vi "RF Scope Control.vi"() -> ()   [LabVIEW 2020]
uses:
  Sub VIs/Scope/Typedefs/Scope Control References Control.ctl
  Sub VIs/Power Supply/Typedefs/Power Supply Models.ctl
  Sub VIs/Settings/Typedefs/Save Settings Control References Control.ctl
  Sub VIs/DMM/Typedefs/DMM Control Variable References.ctl
  Sub VIs/Power Supply/Typedefs/PS Control Variable References.ctl
  Sub VIs/Measurements/Typedefs/Experiment Config Control.ctl
  Sub VIs/Measurements/Typedefs/Measurement Config.ctl
  Sub VIs/Settings/Typedefs/Save settings cluster.ctl
  Sub VIs/Global Vars.vi
  <vilib>/Utility/file.llb/Write Delimited Spreadsheet (string).vi
panel:
  in  "Scope Control References":T1
  in  "PS Reconnecting 2":bool
  in  "DMM Reconnecting 2":bool
  out "Headers":string[](array[string])
  in  "Scope Reconnecting":bool
  in  "PS Reconnecting":bool
  in  "DMM Reconnecting":bool
  in  "Tab Control 2":T2(tab)
  in  "Scope Config on Startup":enum16{"PC->Scope", "Scope->PC"}(ring)=enum."Scope->PC"
  in  "Scope Model":u16(ring)=1 items=["Tek TDS 684A/B/C", "Tek TDS 694C", "Tek TDS 744/A", "Tek TDS 754A/C/D", "Tek TDS 784A/C/D"]
  in  "Disconnect Scope":bool
  in  "Connect Scope":bool
  in  "Reset Settings":bool
  out "Connected Scope":string
  in  "Scope Address":refnum<visa-resource-name>
  out "Scope Connected":bool
  in  "Vertical Scale":u16(ring)=6 items=["1mV", "2mV", "5mV", "10mV", "20mV", "50mV", "100mV", "200mV", "500mV", "1V", "2V", "5V", "10V"]
  in  "Trigger Coupling":i32(ring)=1 items=["main trigger", "DC", "noise reject"]
  in  "Trigger Slope":i32(ring) items=["Positive", "Negative"]
  in  "Horizontle Scale":i32(ring)=19 items=["100ps/div", "200ps/div", "500ps/div", "1ns/div", "2ns/div", "5ns/div", "10ns/div", "20ns/div", "50ns/div", "100ns/div", "200ns/div", "500ns/div", "1µs/div", "2µs/div", "5µs/div", "10µs/div", "20µs/div", "50µs/div", "100µs/div", "200µs/div", "500µs/div", "1ms/div", "2ms/div", "5ms/div", "10ms/div", "20ms/div", "50ms/div", "100ms/div", "200ms/div", "500ms/div", "1s/div", "2s/div", "5s/div", "10s/div"]
  in  "Horizontle Trace Display":i32(ring)=1 items=["Main Only", "Intensified", "Delayed Only"]
  in  "Record Sample Length":i32(ring)=2 items=["500 points", "1000 points", "2500 points", "5000 points", "15000 points", "50000 points", "75000 points", "100000 points", "130000 points", "250000 points", "500000 points"]
  in  "Trigger Source":u16(ring) items=["Ch. 01", "Ch 02", "Ch. 03", "Ch. 04", "Aux"]
  in  "Trigger Level (V)":dbl
  in  "Trigger Type":u16(ring)=1 items=["Auto", "Normal"]
  in  "Coupling":u16(ring)=1 items=["AC", "DC", "Ground"]
  in  "Bandwidth":u16(ring)=2 items=["20 MHz", "250 MHz", "Full"]
  in  "Input Impedance":u16(ring) items=["50 Ohm", "1 MOhm"]
  in  "Waveform Source":u16(ring) items=["Ch. 01", "Ch 02", "Ch. 03", "Ch. 04"]
  in  "Repetitive Signal":bool
  in  "Power Supply Model 2":T3=enum."Keithley 24XX"
  in  "Power Supply Config on Startup 2":enum16{"PC->Power Supply", "Power Supply->PC"}(ring)=enum."Power Supply->PC"
  out "PS Connected 2":bool
  in  "Disconnect PS 2":bool
  in  "Connect PS 2":bool
  in  "ResetPS Settings 2":bool=TRUE
  out "Connected Power Supply 2":string
  in  "Power Supply Address 2":refnum<visa-resource-name>="GPIB0::5::INSTR"
  in  "Power Supply Config on Startup":enum16{"PC->Power Supply", "Power Supply->PC"}(ring)=enum."Power Supply->PC"
  out "PS Connected":bool
  in  "Disconnect PS":bool
  in  "Connect PS":bool
  in  "ResetPS Settings":bool=TRUE
  out "Connected Power Supply":string
  in  "Power Supply Address":refnum<visa-resource-name>="GPIB0::5::INSTR"
  in  "Power Supply Model":T3=enum."Keithley 24XX"
  out "Output Current 2":dbl
  in  "Filter Mode 2":u16(ring) items=["Output Filter Disabled", "Filter 1 On", "Filter 2 On"]
  in  "HV Out 2":bool
  in  "Trip Mode 2":u16(ring) items=["Manual Trip", "Auto Trip"]
  in  "Current Trip 2":dbl=0.005 min=0.0 max=0.005 step=1e-06 format="%.6f"
  in  "Voltage Limit 2":dbl=1000.0
  in  "Current Limit 2":dbl=0.0049 min=0.0 max=0.005 step=1e-06 format="%.6f"
  in  "Voltage Level 2":sgl
  out "Output Voltage 2":dbl
  out "Output Current":dbl
  in  "Filter Mode":u16(ring) items=["Output Filter Disabled", "Filter 1 On", "Filter 2 On"]
  in  "HV Out":bool
  in  "Trip Mode":u16(ring) items=["Manual Trip", "Auto Trip"]
  in  "Current Trip":dbl=0.005 min=0.0 max=0.005 step=1e-06 format="%.6f"
  in  "Voltage Limit":dbl=1000.0
  in  "Current Limit":dbl=0.0049 min=0.0 max=0.005 step=1e-06 format="%.6f"
  in  "Voltage Level":sgl
  out "Output Voltage":dbl
  in  "Identify DMM 2":bool
  in  "Identify DMM":bool
  in  "DMM Config on Startup 2":enum16{"PC->DMM", "DMM->PC"}(ring)=enum."DMM->PC"
  out "DMM Connected 2":bool
  in  "DMM Model 2":u16(ring) items=["Agilent 34405A"]
  in  "Disconnect DMM 2":bool
  in  "Connect DMM 2":bool
  in  "DMM Reset 2":bool
  out "Connected DMM 2":string
  in  "DMM Address 2":refnum<visa-resource-name>="GPIB0::5::INSTR"
  in  "DMM Config on Startup":enum16{"PC->DMM", "DMM->PC"}(ring)=enum."DMM->PC"
  out "DMM Connected":bool
  in  "DMM Model":u16(ring) items=["Agilent 34405A"]
  in  "Disconnect DMM":bool
  in  "Connect DMM":bool
  in  "DMM Reset":bool
  out "Connected DMM":string
  in  "DMM Address":refnum<visa-resource-name>="GPIB0::5::INSTR"
  out "DMM Measurement 2":dbl
  in  "DMM Measurement Type 2":i32(ring) items=["DC Volts", "AC Volts", "DC Current", "AC Current", "2-Wire Resistance", "Frequency", "Temperature", "Capacitance", "Continuity", "Diode", "4-Wire Resistance", "2nd DC Volts", "2nd AC Volts", "2nd DC Current", "2nd AC Current", "2nd Frequency"]
  out "DMM Measurement":dbl
  in  "DMM Measurement Type":i32(ring) items=["DC Volts", "AC Volts", "DC Current", "AC Current", "2-Wire Resistance", "Frequency", "Temperature", "Capacitance", "Continuity", "Diode", "4-Wire Resistance", "2nd DC Volts", "2nd AC Volts", "2nd DC Current", "2nd AC Current", "2nd Frequency"]
  in  "Delimiter":u8(ring)=44 items=["Comma"=44, "Tab"=9, "Semicolon"=59]
  out "Traces Saved":u64
  out "Filename":string
  in  "Start Measurement":bool
  in  "Stop Measurement":bool
  in  "Traces to Acquire":u64=100 min=1 step=1
  in  "Measurement Mode":T4(ring)
  out "Full File Path":path
  out "Measurements Running":bool
  out "Scope Trace":waveform(dbl)(graph)
  in  "Exit":bool
  # "Diode Power Supply"
  # "Amplifier Power Supply"
  # "HV ON"
  # "HV ON"
  # "HV OFF"
  # "HV OFF"
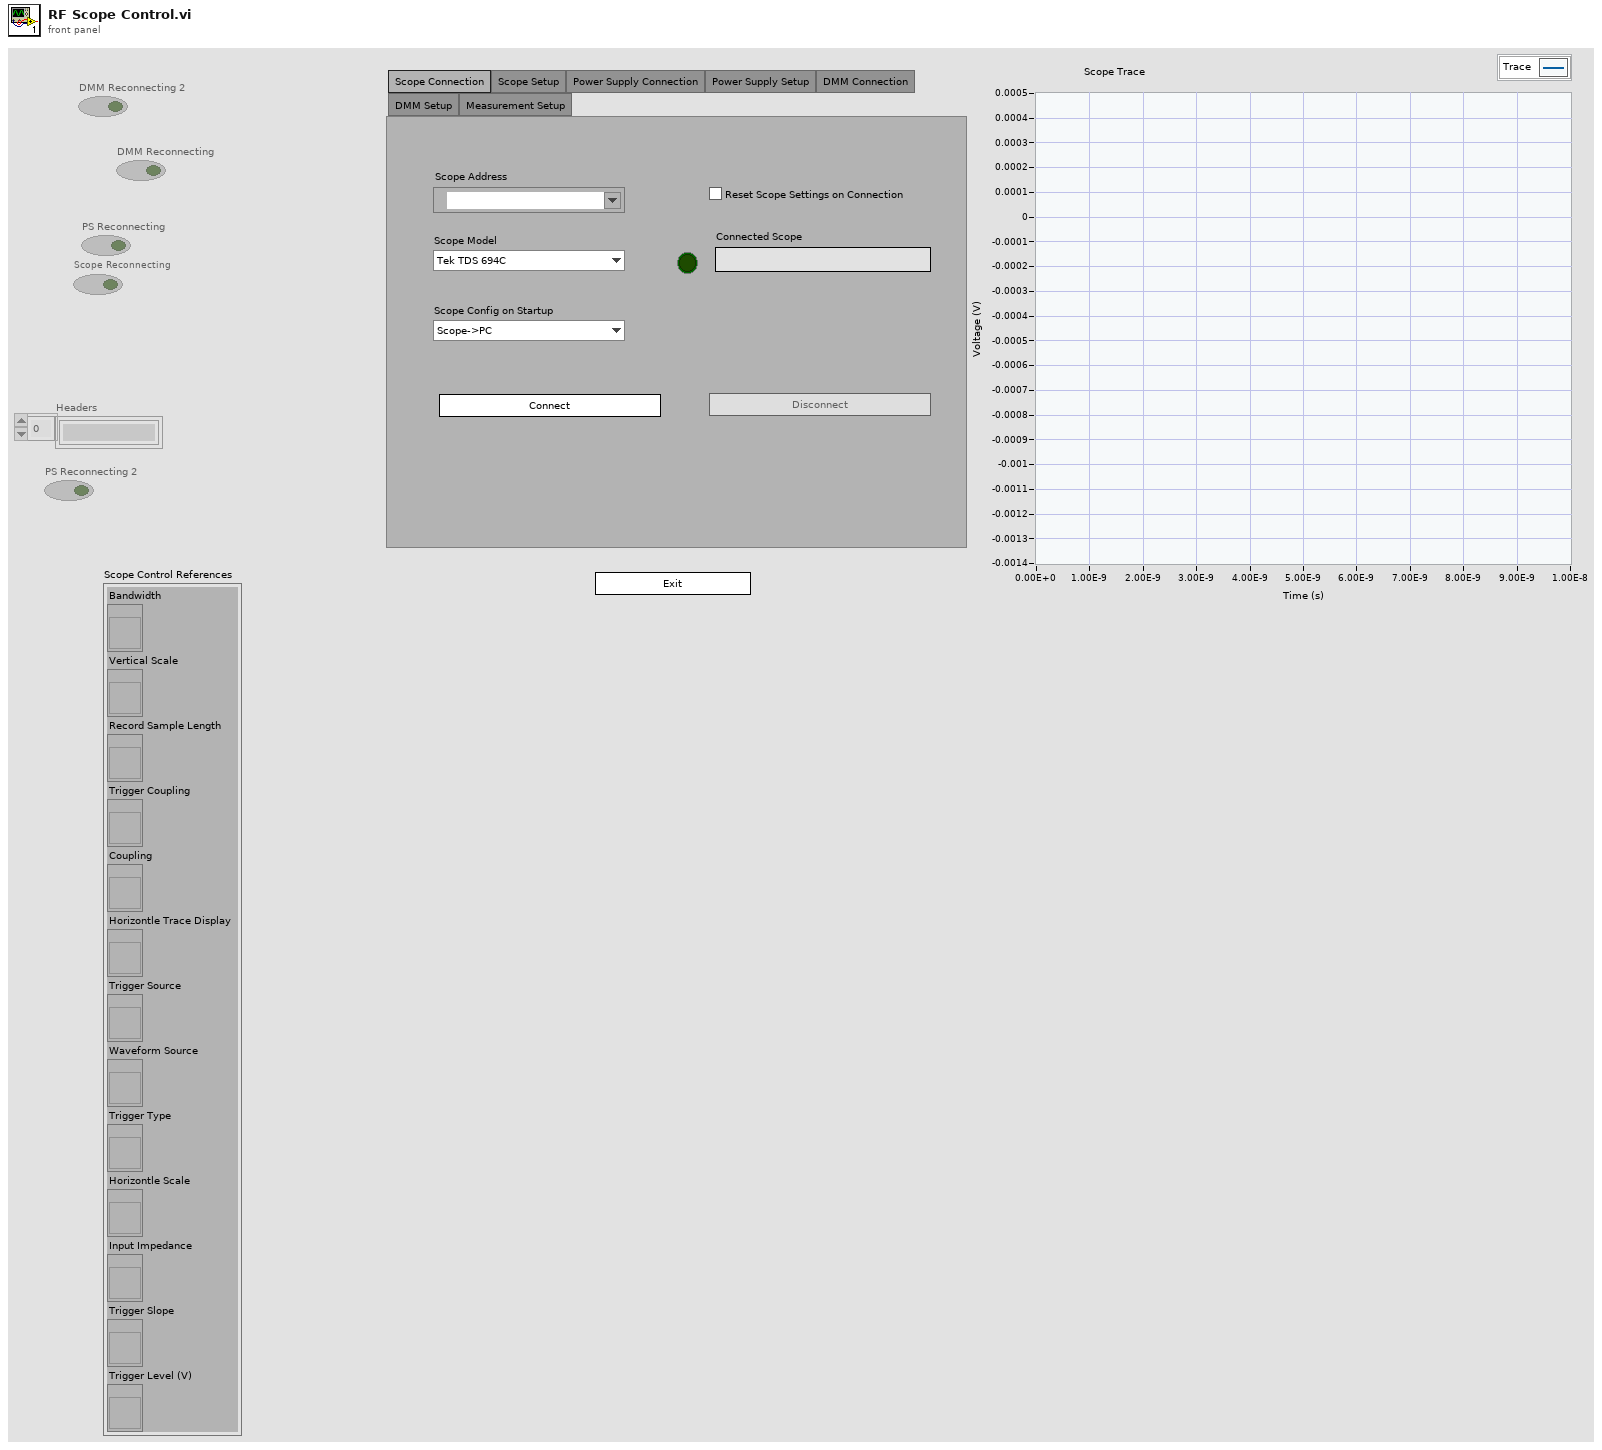
[diagram p1: front panel]
types:
  T1 = typedef "Scope Control References Control.ctl" = cluster{"Bandwidth":refnum<vi>, "Vertical Scale":refnum<vi>, "Record Sample Length":refnum<vi>, "Trigger Coupling":refnum<vi>, "Coupling":refnum<vi>, "Horizontle Trace Display":refnum<vi>, "Trigger Source":refnum<vi>, "Waveform Source":refnum<vi>, "Trigger Type":refnum<vi>, "Horizontle Scale":refnum<vi>, "Input Impedance":refnum<vi>, "Trigger Slope":refnum<vi>, "Trigger Level (V)":refnum<vi>}
  T2 = enum32{"Scope Connection", "Scope Setup", "Power Supply Connection", "Power Supply Setup", "DMM Connection", "DMM Setup", "Measurement Setup"}
  T3 = typedef "Power Supply Models.ctl" = enum16{"Keithley 248", "Keithley 237", "Keithley 24XX", "HP/Agilent 6XXX"}
  T4 = enum16{"Store All Traces in Single File", "Store Average/Std. Dev. for each Point", "Store All Traces in Separate Files"}
  T5 = typedef "PS Control Variable References.ctl" = cluster{"Exit":refnum<vi>, "Power Supply Address":refnum<vi>, "ResetPS Settings":refnum<vi>, "Power Supply Model":refnum<vi>, "PS Connected":refnum<vi>, "Connected Power Supply":refnum<vi>, "Power Supply Config on Startup":refnum<vi>, "Connect PS":refnum<vi>, "Disconnect PS":refnum<vi>, "Voltage Level":refnum<vi>, "Voltage Limit":refnum<vi>, "Current Trip":refnum<vi>, "Current Limit":refnum<vi>, "Trip Mode":refnum<vi>, "Filter Mode":refnum<vi>, "HV Out":refnum<vi>, "Output Voltage":refnum<vi>, "Output Current":refnum<vi>, "PS Reconnecting":refnum<vi>, "semaphore":T6, "Offline Controls":refnum<vi>[], "Online Controls":refnum<vi>[]}
  T6 = typedef "Semaphore RefNum" = refnum<k1>
  T7 = typedef "DMM Control Variable References.ctl" = cluster{"Exit":refnum<vi>, "DMM Connected":refnum<vi>, "DMM Reconnecting":refnum<vi>, "DMM Address":refnum<vi>, "DMM Model":refnum<vi>, "DMM Measurement":refnum<vi>, "Wait on Other Threads":refnum<vi>, "DMM Reset":refnum<vi>, "DMM Config on Startup":refnum<vi>, "DMM Measurement Type":refnum<vi>, "Disconnect DMM":refnum<vi>, "Connect DMM":refnum<vi>, "Identify DMM":refnum<vi>, "Connected DMM":refnum<vi>, "semaphore":T6, "Online Controls":refnum<vi>[], "Offline Controls":refnum<vi>[]}
  T8 = typedef "Save Settings Control References Control.ctl" = cluster{"DMM Config on Startup":refnum<vi>, "Power Supply Config on Startup":refnum<vi>, "Repetitive Signal":refnum<vi>, "Scope Address":refnum<vi>, "Reset Settings":refnum<vi>, "Scope Model":refnum<vi>, "Scope Config on Startup":refnum<vi>, "Waveform Source":refnum<vi>, "Input Impedance":refnum<vi>, "Bandwidth":refnum<vi>, "Coupling":refnum<vi>, "Horizontle Trace Display":refnum<vi>, "Horizontle Scale":refnum<vi>, "Record Sample Length":refnum<vi>, "Trigger Source":refnum<vi>, "Trigger Level (V)":refnum<vi>, "Trigger Slope":refnum<vi>, "Trigger Coupling":refnum<vi>, "Vertical Scale":refnum<vi>, "Trigger Type":refnum<vi>, "Power Supply Address":refnum<vi>, "ResetPS Settings":refnum<vi>, "Voltage Level":refnum<vi>, "Voltage Limit":refnum<vi>, "Current Trip":refnum<vi>, "Current Limit":refnum<vi>, "Trip Mode":refnum<vi>, "Filter Mode":refnum<vi>, "DMM Address":refnum<vi>, "DMM Reset":refnum<vi>, "DMM Model":refnum<vi>, "DMM Measurement Type":refnum<vi>, "Traces to Acquire":refnum<vi>, "Measurement Mode":refnum<vi>, "Power Supply Model":refnum<vi>}
  T9 = enum8{"Enabled", "Disabled", "Disabled and Grayed Out"}
  T10 = typedef "Save settings cluster.ctl" = cluster{"Bandwidth":u16, "Coupling":u16, "Current Limit":dbl, "Current Trip":dbl, "DMM Address":refnum<visa-resource-name>, "DMM Measurement Type":i32, "DMM Model":u16, "DMM Reset":bool, "Filter Mode":u16, "Horizontle Scale":i32, "Horizontle Trace Display":i32, "Input Impedance":u16, "Power Supply Address":refnum<visa-resource-name>, "Record Sample Length":i32, "Reset Settings":bool, "ResetPS Settings":bool, "Scope Address":refnum<visa-resource-name>, "Scope Config on Startup":u16, "Traces to Acquire":u64, "Trigger Coupling":i32, "Trigger Level (V)":dbl, "Trigger Slope":i32, "Trigger Source":u16, "Trigger Type":u16, "Trip Mode":u16, "Vertical Scale":u16, "Voltage Level":sgl, "Voltage Limit":dbl, "Waveform Source":u16, "Scope Model":u16, "DMM Config on Startup":enum16{"PC->DMM", "DMM->PC"}, "Power Supply Config on Startup":enum16{"PC->Power Supply", "Power Supply->PC"}, "Repetitive Signal":bool, "Measurement Mode":enum16{"Store All Traces in Single File", "Store Average/Std. Dev. for each Point", "Store All Traces in Separate Files"}, "Power Supply Model":T3}
  T11 = typedef "Measurement Config.ctl" = cluster{"Measurement Mode":enum16{"Store All Traces in Single File", "Store Average/Std. Dev. for each Point", "Store All Traces in Separate Files"}, "Full File Path":path, "Filename":string, "Delimiter":string, "Headers":string[]}
  T12 = typedef "Experiment Config Control.ctl" = cluster{"PS Connected":bool, "DMM Connected":bool, "DMM Connected 2":bool, "PS HV On":bool}
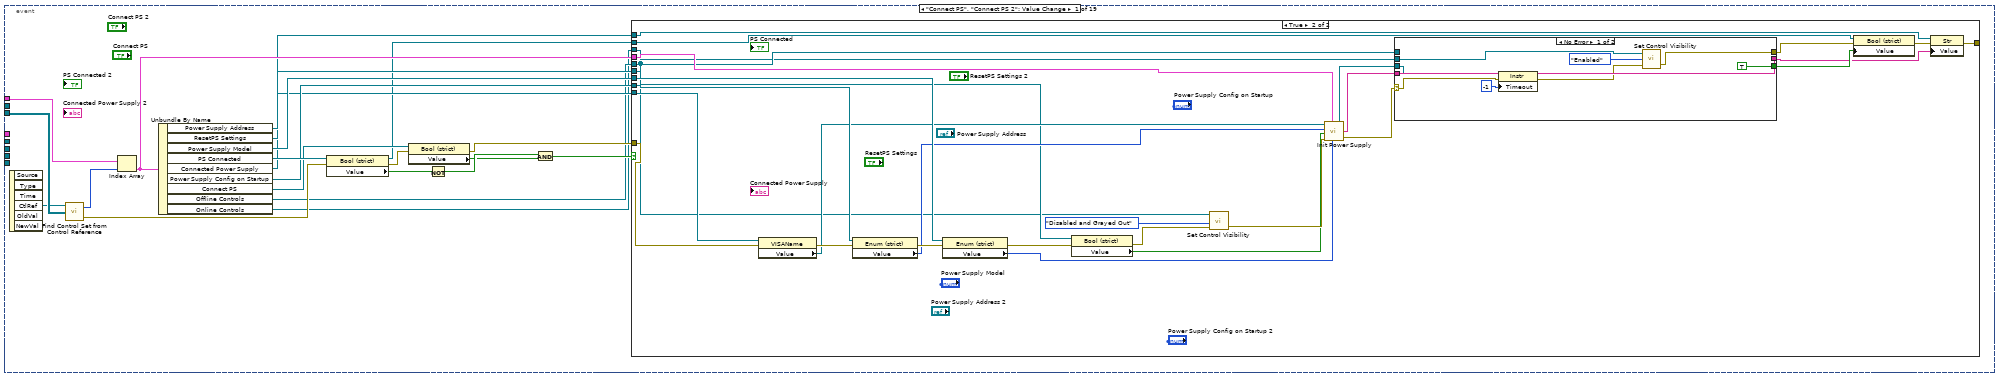
[diagram p14: hidden frame]
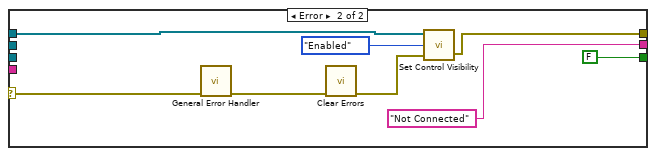
[diagram p16: hidden frame]
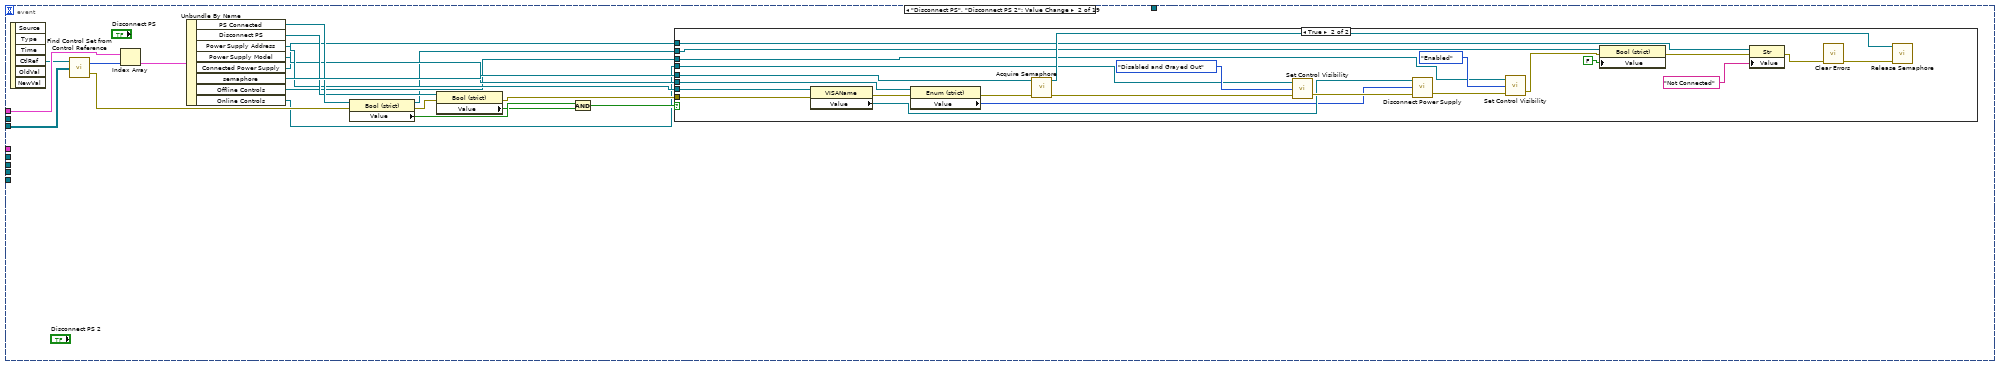
[diagram p17: hidden frame]
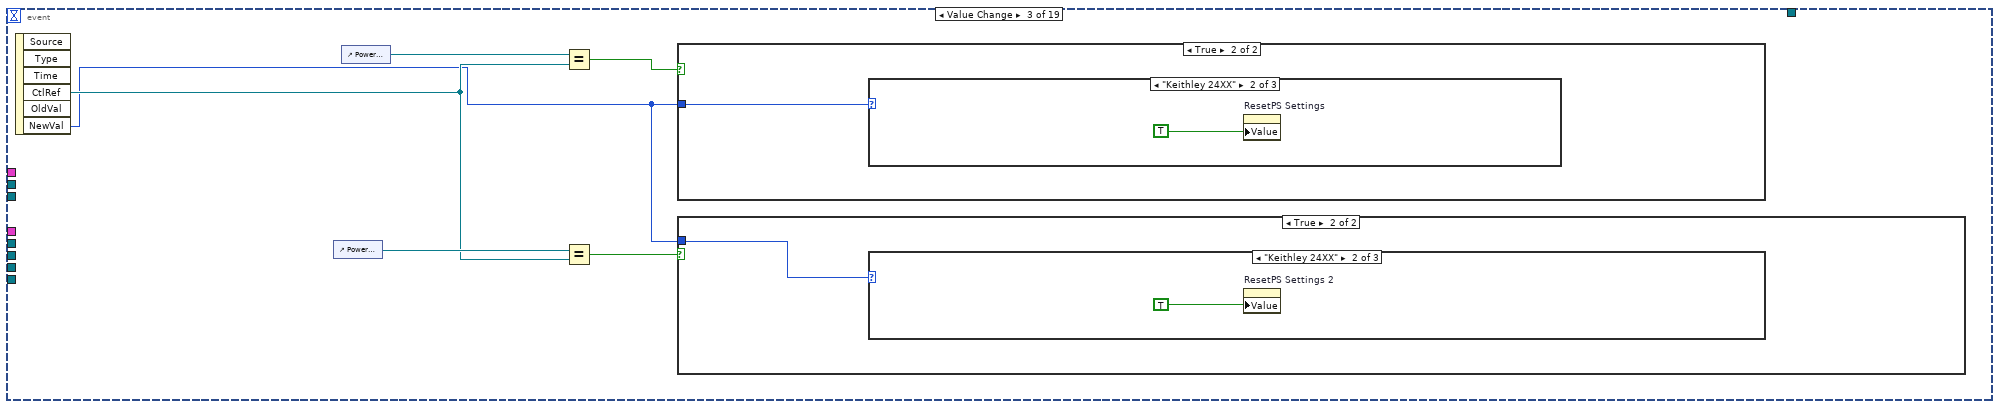
[diagram p19: hidden frame]
diagram:
  w31 = T5 {"Exit"=refnum, "Power Supply Address"=refnum, "ResetPS Settings"=refnum, "Power Supply Model"=refnum, "PS Connected"=refnum, "Connected Power Supply"=refnum, "Power Supply Config on Startup"=refnum, "Connect PS"=refnum, "Disconnect PS"=refnum, "Voltage Level"=refnum, "Voltage Limit"=refnum, "Current Trip"=refnum, "Current Limit"=refnum, "Trip Mode"=refnum, "Filter Mode"=refnum, "HV Out"=refnum, "Output Voltage"=refnum, "Output Current"=refnum, "PS Reconnecting"=refnum, "semaphore"=refnum, "Offline Controls"=[], "Online Controls"=[]}  # PS Control References Array
  w78 = T7 {"Exit"=refnum, "DMM Connected"=refnum, "DMM Reconnecting"=refnum, "DMM Address"=refnum, "DMM Model"=refnum, "DMM Measurement"=refnum, "Wait on Other Threads"=refnum, "DMM Reset"=refnum, "DMM Config on Startup"=refnum, "DMM Measurement Type"=refnum, "Disconnect DMM"=refnum, "Connect DMM"=refnum, "Identify DMM"=refnum, "Connected DMM"=refnum, "semaphore"=refnum, "Online Controls"=[], "Offline Controls"=[]}  # DMM Control References Array
  w112 = T8 {"DMM Config on Startup"=refnum, "Power Supply Config on Startup"=refnum, "Repetitive Signal"=refnum, "Scope Address"=refnum, "Reset Settings"=refnum, "Scope Model"=refnum, "Scope Config on Startup"=refnum, "Waveform Source"=refnum, "Input Impedance"=refnum, "Bandwidth"=refnum, "Coupling"=refnum, "Horizontle Trace Display"=refnum, "Horizontle Scale"=refnum, "Record Sample Length"=refnum, "Trigger Source"=refnum, "Trigger Level (V)"=refnum, "Trigger Slope"=refnum, "Trigger Coupling"=refnum, "Vertical Scale"=refnum, "Trigger Type"=refnum, "Power Supply Address"=refnum, "ResetPS Settings"=refnum, "Voltage Level"=refnum, "Voltage Limit"=refnum, "Current Trip"=refnum, "Current Limit"=refnum, "Trip Mode"=refnum, "Filter Mode"=refnum, "DMM Address"=refnum, "DMM Reset"=refnum, "DMM Model"=refnum, "DMM Measurement Type"=refnum, "Traces to Acquire"=refnum, "Measurement Mode"=refnum, "Power Supply Model"=refnum}  # Controls References
  n1 = control-ref of="Power Supply Config on Startup"() -> (w51:refnum<vi>)
  n2 = control-ref of="DMM Measurement Type"() -> (w83:refnum<vi>)
  n3 = control-ref of="Scope Config on Startup"() -> (w96:refnum<vi>)
  n4 = control-ref of="DMM Config on Startup"() -> (w84:refnum<vi>)
  n5 = control-ref of="Horizontle Trace Display"() -> (w102:refnum<vi>)
  n6 = control-ref of="Power Supply Address"() -> (w53:refnum<vi>)
  n7 = control-ref of="DMM Address"() -> (w88:refnum<vi>)
  n8 = control-ref of="Scope Address"() -> (w109:refnum<vi>)
  n9 = control-ref of="Record Sample Length"() -> (w101:refnum<vi>)
  n10 = control-ref of="Power Supply Model"() -> (w90:refnum<vi>)
  n11 = control-ref of="Power Supply Model"() -> (w50:refnum<vi>)
  n12 = control-ref of="Measurement Mode"() -> (w97:refnum<vi>)
  n13 = control-ref of="Disconnect Scope"() -> (w119:refnum<vi>)
  n14 = control-ref of="Waveform Source"() -> (w107:refnum<vi>)
  n15 = control-ref of="Input Impedance"() -> (w91:refnum<vi>)
  n16 = control-ref of="Traces to Acquire"() -> (w98:refnum<vi>)
  n17 = control-ref of="Trigger Coupling"() -> (w100:refnum<vi>)
  n18 = control-ref of="ResetPS Settings"() -> (w52:refnum<vi>)
  n19 = control-ref of="Repetitive Signal"() -> (w108:refnum<vi>)
  n20 = control-ref of="Horizontle Scale"() -> (w93:refnum<vi>)
  n21 = control-ref of="Trigger Level (V)"() -> (w104:refnum<vi>)
  n22 = control-ref of="Connect Scope"() -> (w118:refnum<vi>)
  n23 = control-ref of="Connect DMM"() -> (w85:refnum<vi>)
  n24 = control-ref of="Trigger Source"() -> (w103:refnum<vi>)
  n25 = control-ref of="Disconnect PS"() -> (w8:refnum<vi>)
  n26 = control-ref of="Reset Settings"() -> (w110:refnum<vi>)
  n27 = control-ref of="Voltage Level"() -> (w47:refnum<vi>)
  n28 = control-ref of="Voltage Limit"() -> (w48:refnum<vi>)
  n29 = control-ref of="Current Limit"() -> (w45:refnum<vi>)
  n30 = control-ref of="Trigger Slope"() -> (w94:refnum<vi>)
  n31 = control-ref of="Vertical Scale"() -> (w99:refnum<vi>)
  n32 = control-ref of="Scope Model"() -> (w95:refnum<vi>)
  n33 = control-ref of="DMM Model"() -> (w87:refnum<vi>)
  n34 = control-ref of="Trigger Type"() -> (w105:refnum<vi>)
  n35 = control-ref of="Current Trip"() -> (w46:refnum<vi>)
  n36 = control-ref of="Connect PS"() -> (w54:refnum<vi>)
  n37 = control-ref of="Filter Mode"() -> (w43:refnum<vi>)
  n38 = control-ref of="DMM Reset"() -> (w89:refnum<vi>)
  n39 = control-ref of="HV Out"() -> (w49:refnum<vi>)
  n40 = control-ref of="Bandwidth"() -> (w92:refnum<vi>)
  n41 = control-ref of="Trip Mode"() -> (w44:refnum<vi>)
  n42 = control-ref of="Coupling"() -> (w106:refnum<vi>)
  n43 = control-ref of="Stop Measurement"() -> (w2:refnum<vi>)
  n44 = Bundle By Name(cluster=w112, "DMM Config on Startup"=w84, "Power Supply Config on Startup"=w51, "Repetitive Signal"=w108, "Scope Address"=w109, "Reset Settings"=w110, "Scope Model"=w95, "Scope Config on Startup"=w96, "Waveform Source"=w107, "Input Impedance"=w91, "Bandwidth"=w92, "Coupling"=w106, "Horizontle Trace Display"=w102, "Horizontle Scale"=w93, "Record Sample Length"=w101, "Trigger Source"=w103, "Trigger Level (V)"=w104, "Trigger Slope"=w94, "Trigger Coupling"=w100, "Vertical Scale"=w99, "Trigger Type"=w105, "Power Supply Address"=w53, "ResetPS Settings"=w52, "Power Supply Model"=w50, "Voltage Level"=w47, "Voltage Limit"=w48, "Current Trip"=w46, "Current Limit"=w45, "Trip Mode"=w44, "Filter Mode"=w43, "DMM Address"=w88, "DMM Reset"=w89, "DMM Model"=w87, "DMM Measurement Type"=w83, "Traces to Acquire"=w98, "Measurement Mode"=w97) -> (w111:T8)
  n45 = Build Array(w119, w107, w106, w105, w103, w104, w94, w102, w101, w100, w93, w99, w108, w92, w91) -> (w130:refnum<vi>[])
  n46 = Build Array(w8, w49, w43, w44, w45, w46, w48, w47) -> (w33:refnum<vi>[])
  n47 = Build Array(w53, w52, w54, w90, w51) -> (w34:refnum<vi>[])
  n48 = Build Array(w88, w89, w85, w84, w87) -> (w62:refnum<vi>[])
  n49 = Build Array(w110, w109, w118, w95, w96) -> (w133:refnum<vi>[])
  n50 = Build Array(w2) -> (w1:refnum<vi>[])
  n51 = Current VI's Path() -> (path=w115:path)
  n52 = call "Recall Settings From XML File.vi"("Controls References"=w111, "Settings File Name"="config.xml", "Settings File Path"=w115) -> ("error out"=w113:errorcluster)  [unwired: 2 in]
  n53 = call <vilib>:"Clear Errors.vi"("error in (no error)"=w113) -> ("error out"=w60:errorcluster)  [unwired: 5 in, 1 out]
  n54 = control-ref of="Disconnect DMM"() -> (w86:refnum<vi>)
  n55 = control-ref of="Identify DMM"() -> (w82:refnum<vi>)
  n56 = Build Array(w86, w83, w82) -> (w61:refnum<vi>[])
  n57 = call <vilib>:"Obtain Semaphore Reference.vi"("error in (no error)"=w60, "name (unnamed)"="DMM Semaphore") -> ("error out"=w137:errorcluster, "semaphore"=w63:T6)  [unwired: 3 in, 1 out]
  n58 = control-ref of="DMM Measurement Type 2"() -> (w72:refnum<vi>)
  n59 = control-ref of="DMM Config on Startup 2"() -> (w76:refnum<vi>)
  n60 = control-ref of="DMM Address 2"() -> (w74:refnum<vi>)
  n61 = control-ref of="DMM Reconnecting 2"() -> (w37:refnum<vi>)
  n62 = control-ref of="DMM Reconnecting"() -> (w80:refnum<vi>)
  n63 = control-ref of="DMM Measurement"() -> (w79:refnum<vi>)
  n64 = control-ref of="Disconnect DMM 2"() -> (w70:refnum<vi>)
  n65 = control-ref of="DMM Connected 2"() -> (w30:refnum<vi>)
  n66 = control-ref of="Start Measurement"() -> (w38:refnum<vi>)
  n67 = control-ref of="PS Reconnecting 2"() -> (w15:refnum<vi>)
  n68 = control-ref of="Connected DMM"() -> (w67:refnum<vi>)
  n69 = control-ref of="DMM Connected"() -> (w81:refnum<vi>)
  n70 = control-ref of="PS Reconnecting"() -> (w35:refnum<vi>)
  n71 = control-ref of="Connect DMM 2"() -> (w73:refnum<vi>)
  n72 = control-ref of="Identify DMM 2"() -> (w71:refnum<vi>)
  n73 = control-ref of="DMM Model 2"() -> (w68:refnum<vi>)
  n74 = control-ref of="PS Connected"() -> (w42:refnum<vi>)
  n75 = control-ref of="DMM Reset 2"() -> (w75:refnum<vi>)
  n76 = control-ref of="HV Out 2"() -> (w18:refnum<vi>)
  n77 = control-ref of="Exit"() -> (w77:refnum<vi>)
  n78 = control-ref of="Measurements Running"() -> (w6:refnum<vi>)
  n79 = control-ref of="Scope Connected"() -> (w7:refnum<vi>)
  n80 = control-ref of="Delimiter"() -> (w4:refnum<vi>)
  n81 = Bundle By Name(cluster=w78, "Exit"=w77, "DMM Connected"=w81, "DMM Reconnecting"=w80, "DMM Address"=w88, "DMM Model"=w87, "DMM Measurement"=w79, "Identify DMM"=w82, "DMM Reset"=w89, "DMM Config on Startup"=w84, "DMM Measurement Type"=w83, "Disconnect DMM"=w86, "Connect DMM"=w85, "Connected DMM"=w67, "semaphore"=w63, "Online Controls"=w61, "Offline Controls"=w62) -> (w64:T7)
  n82 = Build Array(w74, w75, w76, w73, w68) -> (w55:refnum<vi>[])
  n83 = Build Array(w70, w72, w71) -> (w56:refnum<vi>[])
  n84 = Build Array(w98, w38, w97, w4) -> (w3:refnum<vi>[])
  n85 = call <vilib>:"Obtain Semaphore Reference.vi"("error in (no error)"=w137, "name (unnamed)"="DMM 2 Semaphore") -> ("error out"=w136:errorcluster, "semaphore"=w57:T6)  [unwired: 3 in, 1 out]
  n86 = global write "Global Vars.vi" "DMM 1 Controls"(w64) -> ()
  n87 = control-ref of="DMM Measurement 2"() -> (w69:refnum<vi>)
  n88 = control-ref of="Connected DMM 2"() -> (w66:refnum<vi>)
  n89 = Bundle By Name(cluster=w78, "Exit"=w77, "DMM Connected"=w30, "DMM Reconnecting"=w37, "DMM Address"=w74, "DMM Model"=w68, "DMM Measurement"=w69, "Identify DMM"=w71, "DMM Reset"=w75, "DMM Config on Startup"=w76, "DMM Measurement Type"=w72, "Disconnect DMM"=w70, "Connect DMM"=w73, "Connected DMM"=w66, "semaphore"=w57, "Online Controls"=w56, "Offline Controls"=w55) -> (w65:T7)
  n90 = call <vilib>:"Obtain Semaphore Reference.vi"("error in (no error)"=w136, "name (unnamed)"="Scope Semaphore") -> ("error out"=w141:errorcluster, "semaphore"=w140:T6)  [unwired: 3 in, 1 out]
  n91 = global write "Global Vars.vi" "DMM 2 Controls"(w65) -> ()
  n92 = control-ref of="Power Supply Config on Startup 2"() -> (w25:refnum<vi>)
  n93 = control-ref of="Power Supply Address 2"() -> (w29:refnum<vi>)
  n94 = control-ref of="Power Supply Model 2"() -> (w27:refnum<vi>)
  n95 = call <vilib>:"Obtain Semaphore Reference.vi"("error in (no error)"=w141, "name (unnamed)"="PS Semaphore") -> ("error out"=w127:errorcluster, "semaphore"=w40:T6)  [unwired: 3 in, 1 out]
  n96 = control-ref of="ResetPS Settings 2"() -> (w28:refnum<vi>)
  n97 = control-ref of="Connect PS 2"() -> (w10:refnum<vi>)
  n98 = control-ref of="Connected Power Supply 2"() -> (w26:refnum<vi>)
  n99 = control-ref of="Connected Power Supply"() -> (w41:refnum<vi>)
  n100 = Build Array(w29, w28, w27, w25, w10) -> (w11:refnum<vi>[])
  n101 = control-ref of="Connected Scope"() -> (w121:refnum<vi>)
  n102 = control-ref of="Disconnect PS 2"() -> (w9:refnum<vi>)
  n103 = control-ref of="Output Voltage"() -> (w39:refnum<vi>)
  n104 = control-ref of="Output Current"() -> (w36:refnum<vi>)
  n105 = control-ref of="Voltage Level 2"() -> (w24:refnum<vi>)
  n106 = control-ref of="Voltage Limit 2"() -> (w23:refnum<vi>)
  n107 = control-ref of="Current Limit 2"() -> (w21:refnum<vi>)
  n108 = control-ref of="Current Trip 2"() -> (w22:refnum<vi>)
  n109 = control-ref of="Filter Mode 2"() -> (w19:refnum<vi>)
  n110 = control-ref of="Trip Mode 2"() -> (w20:refnum<vi>)
  n111 = Bundle By Name(cluster=w31, "Exit"=w30, "Power Supply Address"=w53, "ResetPS Settings"=w52, "Power Supply Model"=w50, "PS Connected"=w42, "Connected Power Supply"=w41, "Power Supply Config on Startup"=w51, "Connect PS"=w54, "Disconnect PS"=w8, "Voltage Level"=w47, "Voltage Limit"=w48, "Current Trip"=w46, "Current Limit"=w45, "Trip Mode"=w44, "Filter Mode"=w43, "HV Out"=w49, "Output Voltage"=w39, "Output Current"=w36, "PS Reconnecting"=w35, "semaphore"=w40, "Offline Controls"=w34, "Online Controls"=w33) -> (w32:T5)
  n112 = Build Array (concatenate)(w11, w55, w62, w34, w133, w1) -> (w131:refnum<vi>[])
  n113 = Build Array(w121, w41, w26, w67, w66) -> (w120:refnum<vi>[])
  n114 = Build Array(w24, w23, w22, w21, w20, w19, w18, w9) -> (w12:refnum<vi>[])
  n115 = call <vilib>:"Obtain Semaphore Reference.vi"("error in (no error)"=w127, "name (unnamed)"="PS 2 Semaphore") -> ("error out"=w59:errorcluster, "semaphore"=w14:T6)  [unwired: 3 in, 1 out]
  n116 = global write "Global Vars.vi" "Diode Power Supply Controls"(w32) -> ()
  n117 = Build Array (concatenate)(w12, w56, w61, w3, w33, w130, w1) -> (w129:refnum<vi>[])
  n118 = control-ref of="Output Voltage 2"() -> (w17:refnum<vi>)
  n119 = control-ref of="Output Current 2"() -> (w16:refnum<vi>)
  n120 = control-ref of="PS Connected 2"() -> (w5:refnum<vi>)
  n121 = Build Array(w6, w5, w7, w15, w18, w70, w71, w86, w82, w49, w8, w38, w119, w37, w118, w54, w85, w73, w77, w42, w81, w80, w30, w35) -> (w122:refnum<vi>[])
  n122 = Bundle By Name(cluster=w31, "Exit"=w30, "Power Supply Address"=w29, "ResetPS Settings"=w28, "Power Supply Model"=w27, "PS Connected"=w5, "Connected Power Supply"=w26, "Power Supply Config on Startup"=w25, "Connect PS"=w10, "Disconnect PS"=w9, "Voltage Level"=w24, "Voltage Limit"=w23, "Current Trip"=w22, "Current Limit"=w21, "Trip Mode"=w20, "Filter Mode"=w19, "HV Out"=w18, "Output Voltage"=w17, "Output Current"=w16, "PS Reconnecting"=w15, "semaphore"=w14, "Offline Controls"=w11, "Online Controls"=w12) -> (w13:T5)
  n123 = call "Set Control Visibility.vi"("error in"=w59, "Disabled"=T9."Enabled", "Controls Reference Array"=w131) -> ("error out"=w132:errorcluster)  [unwired: 1 in]
  n124 = global write "Global Vars.vi" "Amp Power Supply Controls 2"(w13) -> ()
  n125 = call "Set Control Visibility.vi"("error in"=w132, "Disabled"=T9."Disabled and Grayed Out", "Controls Reference Array"=w129) -> ("error out"=w117:errorcluster)  [unwired: 1 in]
  n126 = To Variant(anything=FALSE) -> (Variant=w125:variant)
  n127 = To Variant(anything="Not Connected") -> (Variant=w123:variant)
  n128 = call "Set Control Value.vi"("error in"=w117, "Value"=w125, "Controls Reference Array"=w122) -> ("error out"=w116:errorcluster)  [unwired: 1 in]
  n129 = call "Set Control Value.vi"("error in"=w116, "Value"=w123, "Controls Reference Array"=w120) -> ("error out"=w58:errorcluster)  [unwired: 1 in]
  n130 = case shown="No Error" w58 {
    selector: w58 -> [_ w1218]
    tunnel: w130 -> [w228 _]
    tunnel: w133 -> [w227 _]
    tunnel: w3 -> [w226 _]
    tunnel: w33 -> [_ _]
    tunnel: w140 -> [w224 _]
    tunnel: [w225 _] -> _
    tunnel: [w222 _] -> _
    tunnel: w1 -> [w144 _]
    frame No Error {
      n131 = while {
        stop <- w234 stop-if-true
        n132 = local read "Exit"() -> (w234:bool)
        n133 = local read "PS Connected 2"() -> (w232:bool)
        n134 = local read "PS Reconnecting 2"() -> (w233:bool)
        n135 = Not(x=w234) -> (.not. x?=w231:bool)
        n136 = Not(x=w233) -> (.not. x?=w230:bool)
        n137 = Compound Arithmetic op=AND(w232, w231, w230) -> (w229:bool)
        n138 = case shown="True" w229 {
          frame False {
          }
          frame True {
            n139 = global read "Global Vars.vi" "Amp Power Supply Controls 2"() -> (w248:T5)
            n140 = Unbundle By Name(w248) -> ("semaphore"=w247:T6, "PS Reconnecting"=w237:refnum<vi>)
            n141 = call <vilib>:"Acquire Semaphore.vi"("semaphore"=w247) -> ("error out"=w245:errorcluster, "semaphore out"=w235:T6)  [unwired: 4 in, 1 out]
            n142 = local read "Power Supply Address 2"() -> (w246:refnum<visa-resource-name>)
            n143 = property class="Instr"(reference=w246, error in=w245, "Timeout"=-1) -> (reference out=w244:refnum<visa-resource-name>, error out=w243:errorcluster)
            n144 = local read "Power Supply Model 2"() -> (w240:T3)
            n145 = call "Get Power Supply Measurement.vi"("Power Supply Address"=w244, "Power Supply Model"=w240, "error in"=w243) -> ("Voltage Output"=→"Output Voltage 2":dbl, "Current Output"=→"Output Current 2":dbl, "error out"=w238:errorcluster)  [unwired: 1 out]
            n146 = call <vilib>:"General Error Handler.vi"("error in (no error)"=w238) -> ("error out"=w239:errorcluster)  [unwired: 10 in, 4 out]
            n147 = case shown="Error .." w239 {
              selector: w239 -> [w250 w255]
              tunnel: [w250 w252] -> w236
              tunnel: w237 -> [_ w251]
              frame No Error {
              }
              frame Error {
                n148 = call <vilib>:"Clear Errors.vi"("error in (no error)"=w255) -> ("error out"=w254:errorcluster)  [unwired: 5 in, 1 out]
                n149 = property on="Property Node" class="Bool (strict)"(reference=w251, error in=w254, "Val(Sgnl)"=TRUE) -> (error out=w252:errorcluster)  [unwired: 1 out]
              }
            }
            n150 = call <vilib>:"Release Semaphore.vi"("error in (no error)"=w236, "semaphore"=w235) -> ()  [unwired: 4 in, 2 out]
          }
        }
      }
      n151 = global read "Global Vars.vi" "Amp Power Supply Controls 2"() -> (w178:T5)
      n152 = global read "Global Vars.vi" "Diode Power Supply Controls"() -> (w217:T5)
      n153 = global read "Global Vars.vi" "DMM 1 Controls"() -> (w197:T7)
      n154 = global read "Global Vars.vi" "DMM 2 Controls"() -> (w149:T7)
      n155 = Unbundle By Name(w178) -> ("Power Supply Address"=w196:refnum<vi>, "ResetPS Settings"=w195:refnum<vi>, "Power Supply Model"=w194:refnum<vi>, "PS Connected"=w193:refnum<vi>, "Connected Power Supply"=w192:refnum<vi>, "Power Supply Config on Startup"=w191:refnum<vi>, "Connect PS"=w190:refnum<vi>, "Disconnect PS"=w189:refnum<vi>, "Voltage Level"=w188:refnum<vi>, "Voltage Limit"=w187:refnum<vi>, "Current Trip"=w186:refnum<vi>, "Current Limit"=w185:refnum<vi>, "Trip Mode"=w184:refnum<vi>, "Filter Mode"=w183:refnum<vi>, "HV Out"=w182:refnum<vi>, "Output Voltage"=w181:refnum<vi>, "Output Current"=w180:refnum<vi>, "PS Reconnecting"=w179:refnum<vi>)
      n156 = Unbundle By Name(w217) -> ("Power Supply Address"=w216:refnum<vi>, "ResetPS Settings"=w215:refnum<vi>, "Power Supply Model"=w214:refnum<vi>, "PS Connected"=w213:refnum<vi>, "Connected Power Supply"=w212:refnum<vi>, "Power Supply Config on Startup"=w211:refnum<vi>, "Connect PS"=w210:refnum<vi>, "Disconnect PS"=w209:refnum<vi>, "Voltage Level"=w208:refnum<vi>, "Voltage Limit"=w207:refnum<vi>, "Current Trip"=w206:refnum<vi>, "Current Limit"=w205:refnum<vi>, "Trip Mode"=w204:refnum<vi>, "Filter Mode"=w203:refnum<vi>, "HV Out"=w202:refnum<vi>, "Output Voltage"=w201:refnum<vi>, "Output Current"=w200:refnum<vi>, "PS Reconnecting"=w199:refnum<vi>)
      n157 = Unbundle By Name(w197) -> ("DMM Connected"=w176:refnum<vi>, "DMM Reconnecting"=w175:refnum<vi>, "DMM Address"=w174:refnum<vi>, "DMM Model"=w173:refnum<vi>, "DMM Measurement"=w172:refnum<vi>, "Wait on Other Threads"=w171:refnum<vi>, "DMM Reset"=w170:refnum<vi>, "DMM Config on Startup"=w169:refnum<vi>, "DMM Measurement Type"=w168:refnum<vi>, "Disconnect DMM"=w167:refnum<vi>, "Connect DMM"=w166:refnum<vi>, "Identify DMM"=w165:refnum<vi>, "Connected DMM"=w164:refnum<vi>)
      n158 = Unbundle By Name(w149) -> ("DMM Connected"=w162:refnum<vi>, "DMM Reconnecting"=w161:refnum<vi>, "DMM Address"=w160:refnum<vi>, "DMM Model"=w159:refnum<vi>, "DMM Measurement"=w158:refnum<vi>, "Wait on Other Threads"=w157:refnum<vi>, "DMM Reset"=w156:refnum<vi>, "DMM Config on Startup"=w155:refnum<vi>, "DMM Measurement Type"=w154:refnum<vi>, "Disconnect DMM"=w153:refnum<vi>, "Connect DMM"=w152:refnum<vi>, "Identify DMM"=w151:refnum<vi>, "Connected DMM"=w150:refnum<vi>)
      n159 = Build Array(w178, w217) -> (w146:T5[])
      n160 = Build Array(w197, w149) -> (w218:T7[])
      n161 = while {
        stop <- w285 stop-if-true
        n162 = local read "DMM Reconnecting"() -> (w282:bool)
        n163 = local read "Exit"() -> (w285:bool)
        n164 = local read "DMM Connected"() -> (w284:bool)
        n165 = Not(x=w285) -> (.not. x?=w283:bool)
        n166 = Not(x=w282) -> (.not. x?=w281:bool)
        n167 = Compound Arithmetic op=AND(w284, w283, w281) -> (w280:bool)
        n168 = case shown="True" w280 {
          frame False {
          }
          frame True {
            n169 = global read "Global Vars.vi" "DMM 1 Controls"() -> (w295:T7)
            n170 = Unbundle By Name(w295) -> ("semaphore"=w294:T6)
            n171 = call <vilib>:"Acquire Semaphore.vi"("semaphore"=w294) -> ("error out"=w296:errorcluster, "semaphore out"=w297:T6)  [unwired: 4 in, 1 out]
            n172 = local read "DMM Address"() -> (w291:refnum<visa-resource-name>)
            n173 = property class="Instr"(reference=w291, error in=w296, "Timeout"=-1) -> (reference out=w290:refnum<visa-resource-name>, error out=w289:errorcluster)
            n174 = local read "DMM Model"() -> (w286:u16)
            n175 = call "Get DMM Measurement.vi"("error in"=w289, "DMM Model"=w286, "DMM Address"=w290) -> ("error out"=w287:errorcluster, "Measurement"=→"DMM Measurement":dbl)  [unwired: 1 out]
            n176 = call <vilib>:"General Error Handler.vi"("error in (no error)"=w287) -> ("error out"=w293:errorcluster)  [unwired: 10 in, 4 out]
            n177 = case shown="Error .." w293 {
              selector: w293 -> [w299 w303]
              tunnel: [w299 w300] -> w298
              frame No Error {
              }
              frame Error {
                n178 = call <vilib>:"Clear Errors.vi"("error in (no error)"=w303) -> ("error out"=w302:errorcluster)  [unwired: 5 in, 1 out]
                n179 = property on="DMM Reconnecting" class="Bool (strict)"(error in=w302, "Val(Sgnl)"=TRUE) -> (error out=w300:errorcluster)  [unwired: 1 in, 1 out]
              }
            }
            n180 = call <vilib>:"Release Semaphore.vi"("error in (no error)"=w298, "semaphore"=w297) -> ()  [unwired: 4 in, 2 out]
          }
        }
      }
      n181 = while {
        stop <- w258 stop-if-true
        n182 = local read "Exit"() -> (w258:bool)
        n183 = local read "DMM Reconnecting 2"() -> (w260:bool)
        n184 = local read "DMM Connected 2"() -> (w257:bool)
        n185 = Not(x=w258) -> (.not. x?=w261:bool)
        n186 = Not(x=w260) -> (.not. x?=w259:bool)
        n187 = Compound Arithmetic op=AND(w261, w259, w257) -> (w256:bool)
        n188 = case shown="True" w256 {
          frame False {
          }
          frame True {
            n189 = global read "Global Vars.vi" "DMM 2 Controls"() -> (w271:T7)
            n190 = Unbundle By Name(w271) -> ("semaphore"=w270:T6)
            n191 = call <vilib>:"Acquire Semaphore.vi"("semaphore"=w270) -> ("error out"=w274:errorcluster, "semaphore out"=w272:T6)  [unwired: 4 in, 1 out]
            n192 = local read "DMM Address 2"() -> (w269:refnum<visa-resource-name>)
            n193 = property class="Instr"(reference=w269, error in=w274, "Timeout"=-1) -> (reference out=w266:refnum<visa-resource-name>, error out=w265:errorcluster)
            n194 = local read "DMM Model 2"() -> (w264:u16)
            n195 = call "Get DMM Measurement.vi"("error in"=w265, "DMM Model"=w264, "DMM Address"=w266) -> ("error out"=w263:errorcluster, "Measurement"=→"DMM Measurement 2":dbl)  [unwired: 1 out]
            n196 = call <vilib>:"General Error Handler.vi"("error in (no error)"=w263) -> ("error out"=w267:errorcluster)  [unwired: 10 in, 4 out]
            n197 = case shown="Error .." w267 {
              selector: w267 -> [w275 w279]
              tunnel: [w275 w276] -> w273
              frame No Error {
              }
              frame Error {
                n198 = call <vilib>:"Clear Errors.vi"("error in (no error)"=w279) -> ("error out"=w277:errorcluster)  [unwired: 5 in, 1 out]
                n199 = property on="DMM Reconnecting 2" class="Bool (strict)"(error in=w277, "Val(Sgnl)"=TRUE) -> (error out=w276:errorcluster)  [unwired: 1 in, 1 out]
              }
            }
            n200 = call <vilib>:"Release Semaphore.vi"("error in (no error)"=w273, "semaphore"=w272) -> ()  [unwired: 4 in, 2 out]
          }
        }
      }
      n201 = while {
        stop <- w306 stop-if-true
        n202 = local read "PS Reconnecting"() -> (w309:bool)
        n203 = local read "Exit"() -> (w306:bool)
        n204 = Not(x=w306) -> (.not. x?=w310:bool)
        n205 = Not(x=w309) -> (.not. x?=w308:bool)
        n206 = local read "PS Connected"() -> (w305:bool)
        n207 = property on="HV Out" class="Bool (strict)"() -> ("Value"=w304:bool)  [unwired: 2 in, 2 out]
        n208 = Compound Arithmetic op=AND(w304, w310, w308, w305) -> (w307:bool)
        n209 = case shown="True" w307 {
          frame False {
          }
          frame True {
            n210 = global read "Global Vars.vi" "Diode Power Supply Controls"() -> (w321:T5)
            n211 = Unbundle By Name(w321) -> ("semaphore"=w320:T6)
            n212 = call <vilib>:"Acquire Semaphore.vi"("semaphore"=w320) -> ("error out"=w322:errorcluster, "semaphore out"=w324:T6)  [unwired: 4 in, 1 out]
            n213 = local read "Power Supply Address"() -> (w317:refnum<visa-resource-name>)
            n214 = property class="Instr"(reference=w317, error in=w322, "Timeout"=-1) -> (reference out=w316:refnum<visa-resource-name>, error out=w315:errorcluster)
            n215 = local read "Power Supply Model"() -> (w311:T3)
            n216 = call "Get Power Supply Measurement.vi"("Power Supply Address"=w316, "Power Supply Model"=w311, "error in"=w315) -> ("Voltage Output"=→"Output Voltage":dbl, "Current Output"=→"Output Current":dbl, "error out"=w314:errorcluster)  [unwired: 1 out]
            n217 = call <vilib>:"General Error Handler.vi"("error in (no error)"=w314) -> ("error out"=w319:errorcluster)  [unwired: 10 in, 4 out]
            n218 = case shown="Error .." w319 {
              selector: w319 -> [w325 w329]
              tunnel: [w325 w326] -> w323
              frame No Error {
              }
              frame Error {
                n219 = call <vilib>:"Clear Errors.vi"("error in (no error)"=w329) -> ("error out"=w327:errorcluster)  [unwired: 5 in, 1 out]
                n220 = property on="PS Reconnecting" class="Bool (strict)"(error in=w327, "Val(Sgnl)"=TRUE) -> (error out=w326:errorcluster)  [unwired: 1 in, 1 out]
              }
            }
            n221 = call <vilib>:"Release Semaphore.vi"("error in (no error)"=w323, "semaphore"=w324) -> ()  [unwired: 4 in, 2 out]
          }
        }
      }
      n222 = while {
        tunnel: w224 -> [w336]
        stop <- w331 stop-if-true
        n223 = local read "Exit"() -> (w331:bool)
        n224 = local read "Scope Reconnecting"() -> (w334:bool)
        n225 = local read "Scope Connected"() -> (w330:bool)
        n226 = Not(x=w331) -> (.not. x?=w335:bool)
        n227 = Not(x=w334) -> (.not. x?=w333:bool)
        n228 = Compound Arithmetic op=AND(w330, w335, w333) -> (w332:bool)
        n229 = case shown="True" w332 {
          tunnel: w336 -> [_ w366]
          frame False {
          }
          frame True {
            n230 = call <vilib>:"Acquire Semaphore.vi"("semaphore"=w366) -> ("error out"=w363:errorcluster, "semaphore out"=w364:T6)  [unwired: 4 in, 1 out]
            n231 = property on="DMM Measurement" class="DigNum (strict)"(error in=w363) -> (error out=w346:errorcluster, "Value"=w352:dbl)  [unwired: 1 in, 1 out]
            n232 = property on="DMM Measurement 2" class="DigNum (strict)"(error in=w346) -> (error out=w345:errorcluster, "Value"=w344:dbl)  [unwired: 1 in, 1 out]
            n233 = property on="Output Voltage" class="DigNum (strict)"(error in=w345) -> (error out=w353:errorcluster, "Value"=w355:dbl)  [unwired: 1 in, 1 out]
            n234 = property on="Output Current" class="DigNum (strict)"(error in=w353) -> (error out=w348:errorcluster, "Value"=w354:dbl)  [unwired: 1 in, 1 out]
            n235 = local read "Scope Address"() -> (w349:refnum<visa-resource-name>)
            n236 = property class="Instr"(reference=w349, error in=w348, "Timeout"=-1) -> (reference out=w342:refnum<visa-resource-name>, error out=w343:errorcluster)
            n237 = local read "Waveform Source"() -> (w337:u16)
            n238 = local read "Scope Model"() -> (w340:u16)
            n239 = call "Get date and time in seconds sequential.vi"("error in (no error)"=w343) -> ("error out"=w341:errorcluster, "current time"=w362:timestamp)  [unwired: 1 in]
            n240 = call "Get Scope Trace.vi"("error in (no error)"=w341, "Waveform Source"=w337, "Scope Model"=w340, "Scope Address"=w342) -> ("error out"=w338:errorcluster, "output waveform"=w339:waveform(dbl))  [unwired: 1 out]
            "Scope Trace" <- w339
            n241 = case shown="Error .." w338 {
              selector: w338 -> [w367 w368]
              tunnel: [w367 w368] -> w350
              frame No Error {
              }
              frame Error {
                n242 = call <vilib>:"Clear Errors.vi"("error in (no error)"=w368) -> ("error out"=w369:errorcluster)  [unwired: 5 in, 1 out]
                n243 = property on="Scope Reconnecting" class="Bool (strict)"(error in=w369, "Val(Sgnl)"=TRUE) -> ()  [unwired: 1 in, 2 out]
              }
            }
            n244 = local read "Traces Saved"() -> (w358:u64)
            n245 = local read "Measurements Running"() -> (w351:bool)
            n246 = Less?(x=w358, y="Traces to Acquire") -> (x < y?=w361:bool)
            n247 = And(x=w361, y=w351) -> (x .and. y?=w360:bool)
            n248 = case shown="True" w360 {
              tunnel: w362 -> [_ w393]
              tunnel: w358 -> [_ w399]
              tunnel: "Traces to Acquire" -> [_ w398]
              tunnel: [w371 w376] -> w357
              tunnel: w350 -> [w371 w395]
              tunnel: w355 -> [_ w391]
              tunnel: w354 -> [_ w392]
              tunnel: w352 -> [_ w389]
              tunnel: w344 -> [_ w390]
              tunnel: w339 -> [_ w394]
              frame False {
              }
              frame True {
                w387 = T11 {"Measurement Mode"=enum."Store All Traces in Single File", "Full File Path"=path "", "Filename"="", "Delimiter"="", "Headers"=[]}  # Measurement Config
                w388 = T12 {"PS Connected"=FALSE, "DMM Connected"=FALSE, "DMM Connected 2"=FALSE, "PS HV On"=FALSE}  # Experiment Config
                n249 = Increment(x=w399) -> (x+1=w396:u64)
                "Traces Saved" <- w396
                n250 = Greater Or Equal?(x=w396, y=w398) -> (x >= y?=w397:bool)
                n251 = local read "DMM Connected 2"() -> (w379:bool)
                n252 = local read "DMM Connected"() -> (w380:bool)
                n253 = local read "PS Connected"() -> (w381:bool)
                n254 = local read "Measurement Mode"() -> (w384:T4)
                n255 = Bundle By Name(cluster=w388, "PS Connected"=w381, "DMM Connected"=w380, "DMM Connected 2"=w379) -> (w378:T12)
                n256 = local read "Delimiter"() -> (w373:u8)
                n257 = local read "Full File Path"() -> (w383:path)
                n258 = local read "Filename"() -> (w385:string)
                n259 = local read "Headers"() -> (w386:string[])
                n260 = Build Array(w373) -> (w375:u8[])
                n261 = Type Cast(type="", x=w375) -> (*(type *) &x=w372:string)
                n262 = Bundle By Name(cluster=w387, "Measurement Mode"=w384, "Full File Path"=w383, "Filename"=w385, "Delimiter"=w372, "Headers"=w386) -> (w382:T11)
                n263 = call "Save Measurement.vi"("Measurement Config"=w382, "Experiment Config"=w378, "DMM Value"=w389, "DMM 2 Value"=w390, "Diode PS Voltage"=w391, "Diode PS Current"=w392, "error in"=w395, "Trace Number"=w396, "Measurement Timestamp"=w393, "Trace"=w394) -> ("error out"=w377:errorcluster)  [unwired: 1 in]
                n264 = case shown="True" w397 {
                  selector: w397 -> [_ w403]
                  tunnel: w377 -> [w400 w401]
                  tunnel: [w400 w401] -> w376
                  frame False {
                  }
                  frame True {
                    n265 = call <vilib>:"Clear Errors.vi"("error in (no error)"=w401) -> ("error out"=w402:errorcluster)  [unwired: 5 in, 1 out]
                    n266 = property on="Stop Measurement" class="Bool (strict)"(error in=w402, "Val(Sgnl)"=w403) -> ()  [unwired: 1 in, 2 out]
                  }
                }
              }
            }
            n267 = call <vilib>:"General Error Handler.vi"("error in (no error)"=w357) -> ("error out"=w356:errorcluster)  [unwired: 10 in, 4 out]
            n268 = call <vilib>:"Clear Errors.vi"("error in (no error)"=w356) -> ("error out"=w365:errorcluster)  [unwired: 5 in, 1 out]
            n269 = call <vilib>:"Release Semaphore.vi"("error in (no error)"=w365, "semaphore"=w364) -> ()  [unwired: 4 in, 2 out]
          }
        }
      }
      n270 = Build Array(w196, w195, w194, w193, w192, w191, w190, w189, w188, w187, w186, w185, w184, w183, w182, w181, w180, w179) -> (w177:refnum<vi>[])
      n271 = Build Array(w216, w215, w214, w213, w212, w211, w210, w209, w208, w207, w206, w205, w204, w203, w202, w201, w200, w199) -> (w198:refnum<vi>[])
      n272 = Build Array(w176, w175, w174, w173, w172, w171, w170, w169, w168, w167, w166, w165, w164) -> (w163:refnum<vi>[])
      n273 = Build Array(w162, w161, w160, w159, w158, w157, w156, w155, w154, w153, w152, w151, w150) -> (w148:refnum<vi>[])
      n274 = Build Array(w177, w198) -> (w145:refnum<vi>[][])
      n275 = Build Array(w163, w148) -> (w147:refnum<vi>[][])
      n276 = while {
        tunnel: w228 -> [w416]
        tunnel: w227 -> [w415]
        tunnel: w226 -> [w414]
        tunnel: w224 -> [w412]
        tunnel: [w411] -> w225
        tunnel: [w410] -> _
        tunnel: [w409] -> w221
        tunnel: w218 -> [w408]
        tunnel: w147 -> [w407]
        tunnel: w146 -> [w406]
        tunnel: w145 -> [w405]
        tunnel: w144 -> [w404]
        stop <- w413 stop-if-true
        n277 = event shown="[16] \"Start Measurement\": Value Change" {
          selector: _ -> [_ _ _ _ _ _ _ _ _ _ _ _ _ _ _ _ _ _ _]
          dyn-events: _ -> [_ _ _ _ _ _ _ _ _ _ _ _ _ _ _ _ _ _ _]
          timeout: _ -> [_ _ _ _ _ _ _ _ _ _ _ _ _ _ _ _ _ _ _]
          tunnel: w416 -> [_ _ _ _ _ w658 w711 _ _ _ _ _ _ _ _ _ _ _ _]
          tunnel: w415 -> [_ _ _ _ _ w657 w712 _ _ _ _ _ _ _ _ _ _ _ _]
          tunnel: w414 -> [_ _ _ _ _ w656 w710 _ _ _ _ _ _ _ _ _ w1053 w1160 _]
          tunnel: [_ _ _ _ _ _ _ _ _ _ _ _ _ _ _ _ _ _ "Exit"] -> w413
          tunnel: w412 -> [_ _ _ _ _ _ w705 w730 w748 w764 w785 _ _ _ _ _ _ _ w1209]
          tunnel: [_ _ _ _ _ _ _ _ _ _ _ _ _ _ _ _ _ _ w1209] -> w411
          tunnel: [_ _ _ _ _ _ _ _ _ _ _ _ _ _ _ _ _ _ w1177] -> w410
          tunnel: [_ _ _ _ _ _ _ _ _ _ _ _ _ _ _ _ _ _ errorcluster {"status"=FALSE, "code"=0, "source"=""} ("error constant")] -> w409
          tunnel: w408 -> [_ _ _ _ _ _ _ _ _ _ _ w830 w896 w939 w967 w999 _ _ _]
          tunnel: w407 -> [_ _ _ _ _ _ _ _ _ _ _ w828 w897 w938 w966 w998 _ _ _]
          tunnel: w406 -> [w435 w501 _ w554 w610 _ _ _ _ _ _ _ _ _ _ _ _ _ _]
          tunnel: w405 -> [w434 w500 _ w556 w612 _ _ _ _ _ _ _ _ _ _ _ _ _ _]
          tunnel: w404 -> [_ _ _ _ _ _ _ _ _ _ _ _ _ _ _ _ w1046 w1156 _]
          event "Connect PS", "Connect PS 2": Value Change {
            n278 = event-data() -> ("CtlRef"=w433:refnum<vi>)  [unwired: 1 in, 5 out]
            n279 = call "Find Control Set from Control Reference.vi"("Control Set Array"=w434, "Control to Search For"=w433) -> ("error out"=w432:errorcluster, "Index"=w436:i32)  [unwired: 1 in]
            n280 = Index Array(array=w435, index=w436) -> (element=w431:T5)
            n281 = Unbundle By Name(w431) -> ("Power Supply Address"=w423:refnum<vi>, "ResetPS Settings"=w421:refnum<vi>, "Power Supply Model"=w425:refnum<vi>, "PS Connected"=w430:refnum<vi>, "Connected Power Supply"=w417:refnum<vi>, "Power Supply Config on Startup"=w424:refnum<vi>, "Connect PS"=w429:refnum<vi>, "Offline Controls"=w420:refnum<vi>[], "Online Controls"=w419:refnum<vi>[])
            n282 = property class="Bool (strict)"(reference=w430, error in=w432) -> (reference out=w418:refnum<vi>, error out=w426:errorcluster, "Value"=w427:bool)
            n283 = property class="Bool (strict)"(reference=w429, error in=w426) -> (error out=w422:errorcluster, "Value"=w428:bool)  [unwired: 1 out]
            n284 = Not(x=w427) -> (.not. x?=w438:bool)
            n285 = And(x=w438, y=w428) -> (x .and. y?=w437:bool)
            n286 = case shown="True" w437 {
              tunnel: [_ w439] -> _
              tunnel: w431 -> [_ w461]
              tunnel: w425 -> [_ w459]
              tunnel: w424 -> [_ w460]
              tunnel: w423 -> [_ w458]
              tunnel: w422 -> [_ w457]
              tunnel: w421 -> [_ w450]
              tunnel: w420 -> [_ w447]
              tunnel: w419 -> [_ w446]
              tunnel: w418 -> [_ w445]
              tunnel: w417 -> [_ w444]
              frame False {
              }
              frame True {
                n287 = property class="VISAName"(reference=w458, error in=w457) -> (error out=w456:errorcluster, "Value"=w454:refnum<visa-resource-name>)  [unwired: 1 out]
                n288 = property class="Enum (strict)"(reference=w460, error in=w456) -> (error out=w455:errorcluster, "Value"=w453:enum16{"PC->Power Supply", "Power Supply->PC"})  [unwired: 1 out]
                n289 = property class="Enum (strict)"(reference=w459, error in=w455) -> (error out=w451:errorcluster, "Value"=w452:T3)  [unwired: 1 out]
                n290 = property class="Bool (strict)"(reference=w450, error in=w451) -> (error out=w448:errorcluster, "Value"=w449:bool)  [unwired: 1 out]
                n291 = call "Set Control Visibility.vi"("error in"=w448, "Disabled"=T9."Disabled and Grayed Out", "Controls Reference Array"=w447) -> ("error out"=w465:errorcluster)  [unwired: 1 in]
                n292 = call "Init Power Supply.vi"("Power Supply Address"=w454, "PS Control References Cluster"=w461, "Power Supply Config on Startup"=w453, "ResetPS Settings"=w449, "Power Supply Model"=w452, "error in"=w465) -> ("VISA resource name out"=w464:refnum<visa-resource-name>, "Instrument Name"=w462:string, "error out"=w463:errorcluster)
                n293 = case shown="No Error" w463 {
                  selector: w463 -> [w469 w482]
                  tunnel: w462 -> [w475 _]
                  tunnel: [w475 "Not Connected"] -> w442
                  tunnel: w464 -> [w470 _]
                  tunnel: [w473 w478] -> w441
                  tunnel: [TRUE ("PS Running") FALSE] -> w443
                  tunnel: w447 -> [_ w476]
                  tunnel: w446 -> [w467 _]
                  frame No Error {
                    n294 = property class="Instr"(reference=w470, error in=w469, "Timeout"=-1) -> (error out=w472:errorcluster)  [unwired: 1 out]
                    n295 = call "Set Control Visibility.vi"("error in"=w472, "Disabled"=T9."Enabled", "Controls Reference Array"=w467) -> ("error out"=w473:errorcluster)  [unwired: 1 in]
                  }
                  frame Error {
                    n296 = call <vilib>:"General Error Handler.vi"("error in (no error)"=w482) -> ("error out"=w481:errorcluster)  [unwired: 10 in, 4 out]
                    n297 = call <vilib>:"Clear Errors.vi"("error in (no error)"=w481) -> ("error out"=w479:errorcluster)  [unwired: 5 in, 1 out]
                    n298 = call "Set Control Visibility.vi"("error in"=w479, "Disabled"=T9."Enabled", "Controls Reference Array"=w476) -> ("error out"=w478:errorcluster)  [unwired: 1 in]
                  }
                }
                n299 = property class="Bool (strict)"(reference=w445, error in=w441, "Value"=w443) -> (error out=w440:errorcluster)  [unwired: 1 out]
                n300 = property class="Str"(reference=w444, error in=w440, "Value"=w442) -> (error out=w439:errorcluster)  [unwired: 1 out]
              }
            }
          }
          event "Disconnect PS", "Disconnect PS 2": Value Change {
            n301 = event-data() -> ("CtlRef"=w499:refnum<vi>)  [unwired: 1 in, 5 out]
            n302 = call "Find Control Set from Control Reference.vi"("Control Set Array"=w500, "Control to Search For"=w499) -> ("error out"=w491:errorcluster, "Index"=w502:i32)  [unwired: 1 in]
            n303 = Index Array(array=w501, index=w502) -> (element=w498:T5)
            n304 = Unbundle By Name(w498) -> ("PS Connected"=w496:refnum<vi>, "Disconnect PS"=w495:refnum<vi>, "Power Supply Address"=w489:refnum<vi>, "Power Supply Model"=w488:refnum<vi>, "Connected Power Supply"=w484:refnum<vi>, "semaphore"=w497:T6, "Offline Controls"=w486:refnum<vi>[], "Online Controls"=w487:refnum<vi>[])
            n305 = property class="Bool (strict)"(reference=w496, error in=w491) -> (reference out=w485:refnum<vi>, error out=w494:errorcluster, "Value"=w493:bool)
            n306 = property class="Bool (strict)"(reference=w495, error in=w494) -> (error out=w490:errorcluster, "Value"=w492:bool)  [unwired: 1 out]
            n307 = And(x=w493, y=w492) -> (x .and. y?=w503:bool)
            n308 = case shown="True" w503 {
              tunnel: w497 -> [_ w520]
              tunnel: w490 -> [_ w519]
              tunnel: w489 -> [_ w517]
              tunnel: w488 -> [_ w516]
              tunnel: w487 -> [_ w513]
              tunnel: w486 -> [_ w512]
              tunnel: w485 -> [_ w510]
              tunnel: w484 -> [_ w507]
              frame False {
              }
              frame True {
                n309 = property class="VISAName"(reference=w517, error in=w519) -> (error out=w518:errorcluster, "Value"=w515:refnum<visa-resource-name>)  [unwired: 1 out]
                n310 = property class="Enum (strict)"(reference=w516, error in=w518) -> (error out=w511:errorcluster, "Value"=w514:T3)  [unwired: 1 out]
                n311 = call <vilib>:"Acquire Semaphore.vi"("error in (no error)"=w511, "semaphore"=w520) -> ("error out"=w523:errorcluster, "semaphore out"=w524:T6)  [unwired: 3 in, 1 out]
                n312 = call "Set Control Visibility.vi"("error in"=w523, "Disabled"=T9."Disabled and Grayed Out", "Controls Reference Array"=w513) -> ("error out"=w526:errorcluster)  [unwired: 1 in]
                n313 = call "Disconnect Power Supply.vi"("error in"=w526, "Power Supply Model"=w514, "Power Supply Address"=w515) -> ("error out"=w521:errorcluster)  [unwired: 1 in]
                n314 = call "Set Control Visibility.vi"("error in"=w521, "Disabled"=T9."Enabled", "Controls Reference Array"=w512) -> ("error out"=w509:errorcluster)  [unwired: 1 in]
                n315 = property class="Bool (strict)"(reference=w510, error in=w509, "Value"=FALSE) -> (error out=w504:errorcluster)  [unwired: 1 out]
                n316 = property class="Str"(reference=w507, error in=w504, "Value"="Not Connected") -> (error out=w505:errorcluster)  [unwired: 1 out]
                n317 = call <vilib>:"Clear Errors.vi"("error in (no error)"=w505) -> ("error out"=w522:errorcluster)  [unwired: 5 in, 1 out]
                n318 = call <vilib>:"Release Semaphore.vi"("error in (no error)"=w522, "semaphore"=w524) -> ()  [unwired: 4 in, 2 out]
              }
            }
          }
          event Value Change {
            n319 = event-data() -> ("CtlRef"=w531:refnum<vi>, "NewVal"=w529:T3)  [unwired: 1 in, 4 out]
            n320 = control-ref of="Power Supply Model 2"() -> (w532:refnum<vi>)
            n321 = control-ref of="Power Supply Model"() -> (w533:refnum<vi>)
            n322 = Equal?(x=w533, y=w531) -> (x = y?=w530:bool)
            n323 = Equal?(x=w532, y=w531) -> (x = y?=w528:bool)
            n324 = case shown="True" w530 {
              tunnel: w529 -> [_ w536]
              frame False {
              }
              frame True {
                n325 = case shown="\"Keithley 24XX\"" w536 {
                  frame "Keithley 248", Default {
                  }
                  frame "Keithley 24XX" {
                    n326 = property on="ResetPS Settings" class="Bool (strict)"("Value"=TRUE) -> ()  [unwired: 2 in, 2 out]
                  }
                  frame "Keithley 237" {
                  }
                }
              }
            }
            n327 = case shown="True" w528 {
              tunnel: w529 -> [_ w534]
              frame False {
              }
              frame True {
                n328 = case shown="\"Keithley 24XX\"" w534 {
                  frame "Keithley 248", Default {
                  }
                  frame "Keithley 24XX" {
                    n329 = property on="ResetPS Settings 2" class="Bool (strict)"("Value"=TRUE) -> ()  [unwired: 2 in, 2 out]
                  }
                  frame "Keithley 237" {
                  }
                }
              }
            }
          }
          event "Filter Mode", "Current Limit", "Voltage Level", "Voltage Limit", "Current Trip", "Trip Mode", "HV Out", "Filter Mode 2", "Current Limit 2", "Voltage Level 2", "Voltage Limit 2", "Current Trip 2", "Trip Mode 2", "HV Out 2": Value Change {
            n330 = event-data() -> ("CtlRef"=w555:refnum<vi>)  [unwired: 1 in, 5 out]
            n331 = call "Find Control Set from Control Reference.vi"("Control Set Array"=w556, "Control to Search For"=w555) -> ("error out"=w550:errorcluster, "Index"=w557:i32)  [unwired: 1 in]
            n332 = Index Array(array=w554, index=w557) -> (element=w553:T5)
            n333 = Unbundle By Name(w553) -> ("PS Connected"=w551:refnum<vi>, "Power Supply Address"=w547:refnum<vi>, "Voltage Level"=w546:refnum<vi>, "Current Limit"=w545:refnum<vi>, "Power Supply Model"=w544:refnum<vi>, "Connected Power Supply"=w543:refnum<vi>, "Current Trip"=w542:refnum<vi>, "HV Out"=w541:refnum<vi>, "Filter Mode"=w540:refnum<vi>, "Trip Mode"=w539:refnum<vi>, "Voltage Limit"=w538:refnum<vi>, "semaphore"=w552:T6)
            n334 = property class="Bool (strict)"(reference=w551, error in=w550) -> (error out=w548:errorcluster, "Value"=w549:bool)  [unwired: 1 out]
            n335 = case shown="True" w549 {
              tunnel: w552 -> [_ w589]
              tunnel: w548 -> [_ w588]
              tunnel: w547 -> [_ w577]
              tunnel: w546 -> [_ w575]
              tunnel: w545 -> [_ w574]
              tunnel: w544 -> [_ w573]
              tunnel: w543 -> [_ w572]
              tunnel: w542 -> [_ w571]
              tunnel: w541 -> [_ w570]
              tunnel: w540 -> [_ w569]
              tunnel: w539 -> [_ w568]
              tunnel: w538 -> [_ w567]
              frame False {
              }
              frame True {
                n336 = property class="VISAName"(reference=w577, error in=w588) -> (error out=w587:errorcluster, "Value"=w576:refnum<visa-resource-name>)  [unwired: 1 out]
                n337 = property class="DigNum (strict)"(reference=w575, error in=w587) -> (error out=w586:errorcluster, "Value"=w566:sgl)  [unwired: 1 out]
                n338 = property class="DigNum (strict)"(reference=w574, error in=w586) -> (error out=w585:errorcluster, "Value"=w565:dbl)  [unwired: 1 out]
                n339 = property class="Enum (strict)"(reference=w573, error in=w585) -> (error out=w584:errorcluster, "Value"=w564:T3)  [unwired: 1 out]
                n340 = property class="Str"(reference=w572, error in=w584) -> (error out=w583:errorcluster, "Value"=w563:string)  [unwired: 1 out]
                n341 = property class="DigNum (strict)"(reference=w571, error in=w583) -> (error out=w582:errorcluster, "Value"=w562:dbl)  [unwired: 1 out]
                n342 = property class="Bool (strict)"(reference=w570, error in=w582) -> (error out=w581:errorcluster, "Value"=w561:bool)  [unwired: 1 out]
                n343 = property class="Ring (strict)"(reference=w569, error in=w581) -> (error out=w580:errorcluster, "Value"=w560:u16)  [unwired: 1 out]
                n344 = property class="Ring (strict)"(reference=w568, error in=w580) -> (error out=w579:errorcluster, "Value"=w559:u16)  [unwired: 1 out]
                n345 = property class="DigNum (strict)"(reference=w567, error in=w579) -> (error out=w578:errorcluster, "Value"=w558:dbl)  [unwired: 1 out]
                n346 = call <vilib>:"Acquire Semaphore.vi"("error in (no error)"=w578, "semaphore"=w589) -> ("error out"=w595:errorcluster, "semaphore out"=w597:T6)  [unwired: 3 in, 1 out]
                n347 = property class="Instr"(reference=w576, error in=w595, "Timeout"=-1) -> (reference out=w593:refnum<visa-resource-name>, error out=w594:errorcluster)
                n348 = call "Update Power Supply Settings.vi"("Power Supply Address"=w593, "Filter Mode"=w560, "Trip Mode"=w559, "Voltage Limit"=w558, "Instrument Name"=w563, "Voltage Level"=w566, "HV Out"=w561, "error in"=w594, "Current Limit"=w565, "Power Supply Model"=w564, "Current Trip"=w562) -> ("error out"=w592:errorcluster)  [unwired: 3 in, 1 out]
                n349 = call <vilib>:"General Error Handler.vi"("error in (no error)"=w592) -> ("error out"=w591:errorcluster)  [unwired: 10 in, 4 out]
                n350 = call <vilib>:"Clear Errors.vi"("error in (no error)"=w591) -> ("error out"=w590:errorcluster)  [unwired: 5 in, 1 out]
                n351 = call <vilib>:"Release Semaphore.vi"("error in (no error)"=w590, "semaphore"=w597) -> ()  [unwired: 4 in, 2 out]
              }
            }
          }
          event "PS Reconnecting": Value Change {
            n352 = event-data() -> ("CtlRef"=w611:refnum<vi>)  [unwired: 1 in, 5 out]
            n353 = call "Find Control Set from Control Reference.vi"("Control Set Array"=w612, "Control to Search For"=w611) -> ("error out"=w600:errorcluster, "Index"=w613:i32)  [unwired: 1 in]
            n354 = Index Array(array=w610, index=w613) -> (element=w609:T5)
            n355 = Unbundle By Name(w609) -> ("PS Connected"=w607:refnum<vi>, "PS Reconnecting"=w606:refnum<vi>, "Power Supply Address"=w602:refnum<vi>, "semaphore"=w608:T6, "Disconnect PS"=w601:refnum<vi>)
            n356 = property class="Bool (strict)"(reference=w607, error in=w600) -> (error out=w599:errorcluster, "Value"=w605:bool)  [unwired: 1 out]
            n357 = property class="Bool (strict)"(reference=w606, error in=w599) -> (error out=w598:errorcluster, "Value"=w604:bool)  [unwired: 1 out]
            n358 = And(x=w605, y=w604) -> (x .and. y?=w603:bool)
            n359 = case shown="True" w603 {
              tunnel: w608 -> [_ w619]
              tunnel: w602 -> [_ w618]
              tunnel: w601 -> [_ w616]
              tunnel: w598 -> [_ w615]
              frame False {
              }
              frame True {
                n360 = property class="VISAName"(reference=w618, error in=w615) -> (error out=w614:errorcluster, "Value"=w617:refnum<visa-resource-name>)  [unwired: 1 out]
                n361 = call <vilib>:"Acquire Semaphore.vi"("error in (no error)"=w614, "semaphore"=w619) -> ("error out"=w623:errorcluster, "semaphore out"=w629:T6)  [unwired: 3 in, 1 out]
                n362 = property class="Instr"(reference=w617, error in=w623, "Timeout"=u32 2000 ("General Settings:Timeout Value")) -> (reference out=w621:refnum<visa-resource-name>, error out=w622:errorcluster)
                n363 = VISA Write(VISA resource name=w621, write buffer="*IDN?" ("ID query"), error in (no error)=w622) -> (VISA resource name out=w626:refnum<visa-resource-name>, error out=w627:errorcluster)  [unwired: 1 out]
                n364 = VISA Read(VISA resource name=w626, byte count=u32 1024, error in (no error)=w627) -> (error out=w625:errorcluster)  [unwired: 3 out]
                n365 = case shown="Error .." w625 {
                  selector: w625 -> [w634 w644]
                  tunnel: [w633 w641] -> w630
                  tunnel: w629 -> [w632 w642]
                  tunnel: w616 -> [_ w636]
                  frame No Error {
                    n366 = call <vilib>:"Release Semaphore.vi"("error in (no error)"=w634, "semaphore"=w632) -> ("error out"=w633:errorcluster)  [unwired: 4 in, 1 out]
                  }
                  frame Error {
                    n367 = call <vilib>:"Clear Errors.vi"("error in (no error)"=w644) -> ("error out"=w643:errorcluster)  [unwired: 5 in, 1 out]
                    n368 = call <vilib>:"Release Semaphore.vi"("error in (no error)"=w643, "semaphore"=w642) -> ("error out"=w637:errorcluster)  [unwired: 4 in, 1 out]
                    n369 = property class="Bool (strict)"(reference=w636, error in=w637, "Val(Sgnl)"=TRUE) -> (error out=w635:errorcluster)  [unwired: 1 out]
                    n370 = property on="Measurements Running" class="Bool (strict)"(error in=w635) -> (error out=w640:errorcluster, "Value"=w639:bool)  [unwired: 1 in, 1 out]
                    n371 = case shown="True" w639 {
                      tunnel: w640 -> [w645 w650]
                      tunnel: [w645 w647] -> w641
                      frame False {
                      }
                      frame True {
                        n372 = call "Display Message to User2"("error in (no error)"=w650, "Message"="Power supply disconnected, stopping measurements.") -> ("error out"=w648:errorcluster)  [unwired: 8 in, 1 out]
                        n373 = property on="Stop Measurement" class="Bool (strict)"(error in=w648, "Val(Sgnl)"=TRUE) -> (error out=w647:errorcluster)  [unwired: 1 in, 1 out]
                      }
                    }
                  }
                }
                n374 = property on="PS Reconnecting" class="Bool (strict)"(error in=w630, "Value"=FALSE) -> ()  [unwired: 1 in, 2 out]
              }
            }
          }
          event "Connect Scope": Value Change {
            n375 = event-data() -> ()  [unwired: 1 in, 6 out]
            n376 = local read "Scope Connected"() -> (w652:bool)
            n377 = Not(x=w652) -> (.not. x?=w651:bool)
            n378 = And(x=w651, y="Connect Scope") -> (x .and. y?=w655:bool)
            n379 = case shown="True" w655 {
              tunnel: w658 -> [_ w688]
              tunnel: w657 -> [_ w684]
              tunnel: w656 -> [_ w686]
              tunnel: [_ FALSE] -> w653
              frame False {
              }
              frame True {
                n380 = control-ref of="Horizontle Trace Display"() -> (w668:refnum<vi>)
                n381 = control-ref of="Record Sample Length"() -> (w666:refnum<vi>)
                n382 = control-ref of="Waveform Source"() -> (w672:refnum<vi>)
                n383 = control-ref of="Input Impedance"() -> (w671:refnum<vi>)
                n384 = control-ref of="Trigger Coupling"() -> (w661:refnum<vi>)
                n385 = control-ref of="Horizontle Scale"() -> (w667:refnum<vi>)
                n386 = control-ref of="Trigger Level (V)"() -> (w663:refnum<vi>)
                n387 = control-ref of="Trigger Source"() -> (w664:refnum<vi>)
                n388 = control-ref of="Vertical Scale"() -> (w660:refnum<vi>)
                n389 = control-ref of="Trigger Slope"() -> (w662:refnum<vi>)
                n390 = control-ref of="Trigger Type"() -> (w665:refnum<vi>)
                n391 = control-ref of="Bandwidth"() -> (w670:refnum<vi>)
                n392 = control-ref of="Coupling"() -> (w669:refnum<vi>)
                n393 = Bundle By Name(cluster="Scope Control References", "Bandwidth"=w670, "Vertical Scale"=w660, "Record Sample Length"=w666, "Trigger Coupling"=w661, "Coupling"=w669, "Horizontle Trace Display"=w668, "Trigger Source"=w664, "Waveform Source"=w672, "Trigger Type"=w665, "Horizontle Scale"=w667, "Input Impedance"=w671, "Trigger Slope"=w662, "Trigger Level (V)"=w663) -> (w675:T1)
                n394 = call "Set Control Visibility.vi"("Disabled"=T9."Disabled and Grayed Out", "Controls Reference Array"=w684) -> ("error out"=w673:errorcluster)  [unwired: 2 in]
                n395 = call "Init Scope.vi"("Timeout (ms)"=u32 2000, "Scope Control References"=w675, "Repetitive Signal"="Repetitive Signal", "Reset Settings"="Reset Settings", "error in (no error)"=w673, "Scope Config on Startup"="Scope Config on Startup", "Scope Model"="Scope Model", "Scope Address"="Scope Address") -> ("error out"=w674:errorcluster, "Instrument ID"=w659:string)  [unwired: 1 out]
                n396 = case shown="No Error" w674 {
                  selector: w674 -> [w692 w703]
                  tunnel: [w691 "Not connected"] -> w689
                  tunnel: w688 -> [w699 _]
                  tunnel: w684 -> [w698 w702]
                  tunnel: [w696 w703] -> w687
                  tunnel: w686 -> [w695 _]
                  tunnel: w659 -> [w691 _]
                  frame No Error {
                    w690 = T9."Enabled" ("Disabled")
                    n397 = call "Set Control Visibility.vi"("error in"=w692, "Disabled"=w690, "Controls Reference Array"=w699) -> ("error out"=w700:errorcluster)  [unwired: 1 in]
                    n398 = call "Set Control Visibility.vi"("error in"=w700, "Disabled"=T9."Disabled and Grayed Out", "Controls Reference Array"=w698) -> ("error out"=w697:errorcluster)  [unwired: 1 in]
                    n399 = call "Set Control Visibility.vi"("error in"=w697, "Disabled"=w690, "Controls Reference Array"=w695) -> ("error out"=w696:errorcluster)  [unwired: 1 in]
                    "Scope Connected" <- TRUE
                  }
                  frame Error {
                    n400 = call "Set Control Visibility.vi"("Disabled"=T9."Enabled", "Controls Reference Array"=w702) -> ()  [unwired: 2 in, 1 out]
                  }
                }
                "Connected Scope" <- w689
                n401 = call <vilib>:"Simple Error Handler.vi"("error in (no error)"=w687) -> ()  [unwired: 4 in, 5 out]
              }
            }
            n402 = property on="Connect Scope" class="Bool (strict)"("Value"=w653) -> ()  [unwired: 2 in, 2 out]
          }
          event "Disconnect Scope": Value Change {
            n403 = event-data() -> ()  [unwired: 1 in, 6 out]
            n404 = local read "Scope Connected"() -> (w708:bool)
            n405 = And(x="Disconnect Scope", y=w708) -> (x .and. y?=w707:bool)
            n406 = case shown="True" w707 {
              tunnel: w712 -> [_ w728]
              tunnel: w711 -> [_ w726]
              tunnel: w710 -> [_ w722]
              tunnel: [_ w721] -> w706
              tunnel: w705 -> [_ w719]
              frame False {
              }
              frame True {
                w721 = FALSE
                w723 = T9."Disabled and Grayed Out" ("Disabled")
                n407 = local read "Scope Address"() -> (w715:refnum<visa-resource-name>)
                n408 = local read "Scope Model"() -> (w713:u16)
                n409 = call <vilib>:"Acquire Semaphore.vi"("semaphore"=w719) -> ("error out"=w716:errorcluster, "semaphore out"=w718:T6)  [unwired: 4 in, 1 out]
                n410 = call "Disconnect Scope.vi"("error in (no error)"=w716, "Scope Model"=w713, "Scope Address"=w715) -> ("error out"=w714:errorcluster)  [unwired: 1 in]
                n411 = call "Set Control Visibility.vi"("error in"=w714, "Disabled"=T9."Enabled", "Controls Reference Array"=w728) -> ("error out"=w729:errorcluster)  [unwired: 1 in]
                n412 = call "Set Control Visibility.vi"("error in"=w729, "Disabled"=w723, "Controls Reference Array"=w726) -> ("error out"=w725:errorcluster)  [unwired: 1 in]
                n413 = call "Set Control Visibility.vi"("error in"=w725, "Disabled"=w723, "Controls Reference Array"=w722) -> ("error out"=w724:errorcluster)  [unwired: 1 in]
                n414 = local write "Scope Connected"(w721) -> ()
                n415 = call <vilib>:"Simple Error Handler.vi"("error in (no error)"=w724) -> ("error out"=w720:errorcluster)  [unwired: 4 in, 4 out]
                n416 = call <vilib>:"Clear Errors.vi"("error in (no error)"=w720) -> ("error out"=w717:errorcluster)  [unwired: 5 in, 1 out]
                n417 = call <vilib>:"Release Semaphore.vi"("error in (no error)"=w717, "semaphore"=w718) -> ()  [unwired: 4 in, 2 out]
              }
            }
            n418 = property on="Disconnect Scope" class="Bool (strict)"("Value"=w706) -> ()  [unwired: 2 in, 2 out]
          }
          event "Coupling", "Bandwidth", "Input Impedance", "Waveform Source", "Vertical Scale": Value Change {
            n419 = event-data() -> ()  [unwired: 1 in, 6 out]
            n420 = local read "Scope Connected"() -> (w731:bool)
            n421 = case shown="True" w731 {
              tunnel: w730 -> [_ w746]
              frame False {
              }
              frame True {
                n422 = local read "Scope Address"() -> (w742:refnum<visa-resource-name>)
                n423 = call <vilib>:"Acquire Semaphore.vi"("semaphore"=w746) -> ("error out"=w741:errorcluster, "semaphore out"=w744:T6)  [unwired: 4 in, 1 out]
                n424 = property class="Instr"(reference=w742, error in=w741, "Timeout"=-1) -> (reference out=w733:refnum<visa-resource-name>, error out=w740:errorcluster)
                n425 = local read "Scope Model"() -> (w732:u16)
                n426 = call "Config Channel.vi"("Scope Model"=w732, "Coupling"="Coupling", "Bandwidth"="Bandwidth", "Input Impedance"="Input Impedance", "error in (no error)"=w740, "Vertical Scale"="Vertical Scale", "Channel"="Waveform Source", "Scope Address"=w733) -> ("error out"=w739:errorcluster)  [unwired: 1 in, 1 out]
                n427 = call <vilib>:"Simple Error Handler.vi"("error in (no error)"=w739) -> ("error out"=w747:errorcluster)  [unwired: 4 in, 4 out]
                n428 = call <vilib>:"Clear Errors.vi"("error in (no error)"=w747) -> ("error out"=w745:errorcluster)  [unwired: 5 in, 1 out]
                n429 = call <vilib>:"Release Semaphore.vi"("error in (no error)"=w745, "semaphore"=w744) -> ()  [unwired: 4 in, 2 out]
              }
            }
          }
          event "Record Sample Length", "Horizontle Trace Display", "Horizontle Scale": Value Change {
            n430 = event-data() -> ()  [unwired: 1 in, 6 out]
            n431 = local read "Scope Connected"() -> (w749:bool)
            n432 = case shown="True" w749 {
              tunnel: w748 -> [_ w761]
              frame False {
              }
              frame True {
                n433 = local read "Scope Address"() -> (w758:refnum<visa-resource-name>)
                n434 = call <vilib>:"Acquire Semaphore.vi"("semaphore"=w761) -> ("error out"=w759:errorcluster, "semaphore out"=w760:T6)  [unwired: 4 in, 1 out]
                n435 = property class="Instr"(reference=w758, error in=w759, "Timeout"=-1) -> (reference out=w755:refnum<visa-resource-name>, error out=w756:errorcluster)
                n436 = local read "Scope Model"() -> (w750:u16)
                n437 = call "Config Horiz.vi"("Scope Model"=w750, "Record Sample Length"="Record Sample Length", "error in (no error)"=w756, "Horizontle Trace Display"="Horizontle Trace Display", "Horizontle Scale"="Horizontle Scale", "Scope Address"=w755) -> ("error out"=w754:errorcluster)  [unwired: 3 in, 1 out]
                n438 = call <vilib>:"General Error Handler.vi"("error in (no error)"=w754) -> ("error out"=w763:errorcluster)  [unwired: 10 in, 4 out]
                n439 = call <vilib>:"Clear Errors.vi"("error in (no error)"=w763) -> ("error out"=w762:errorcluster)  [unwired: 5 in, 1 out]
                n440 = call <vilib>:"Release Semaphore.vi"("error in (no error)"=w762, "semaphore"=w760) -> ()  [unwired: 4 in, 2 out]
              }
            }
          }
          event "Trigger Type", "Trigger Source", "Trigger Level (V)", "Trigger Slope", "Trigger Coupling": Value Change {
            n441 = event-data() -> ()  [unwired: 1 in, 6 out]
            n442 = local read "Scope Connected"() -> (w765:bool)
            n443 = case shown="True" w765 {
              tunnel: w764 -> [_ w781]
              frame False {
              }
              frame True {
                n444 = local read "Scope Address"() -> (w777:refnum<visa-resource-name>)
                n445 = call <vilib>:"Acquire Semaphore.vi"("semaphore"=w781) -> ("error out"=w776:errorcluster, "semaphore out"=w779:T6)  [unwired: 4 in, 1 out]
                n446 = property class="Instr"(reference=w777, error in=w776, "Timeout"=-1) -> (reference out=w773:refnum<visa-resource-name>, error out=w774:errorcluster)
                n447 = local read "Scope Model"() -> (w766:u16)
                n448 = call "Config Trigger.vi"("Scope Model"=w766, "Trigger Coupling"="Trigger Coupling", "Trigger Slope"="Trigger Slope", "Trigger Level (V)"="Trigger Level (V)", "error in (no error)"=w774, "Trigger Source"="Trigger Source", "Trigger Type"="Trigger Type", "Scope Address"=w773) -> ("error out"=w767:errorcluster)  [unwired: 1 in, 1 out]
                n449 = case shown="Error .." w767 {
                  selector: w767 -> [w783 w784]
                  tunnel: [w783 w784] -> w778
                  frame No Error {
                  }
                  frame Error {
                    n450 = call "Display Message to User5"() -> ()  [unwired: 10 in, 2 out]
                  }
                }
                n451 = call <vilib>:"Simple Error Handler.vi"("error in (no error)"=w778) -> ("error out"=w782:errorcluster)  [unwired: 4 in, 4 out]
                n452 = call <vilib>:"Clear Errors.vi"("error in (no error)"=w782) -> ("error out"=w780:errorcluster)  [unwired: 5 in, 1 out]
                n453 = call <vilib>:"Release Semaphore.vi"("error in (no error)"=w780, "semaphore"=w779) -> ()  [unwired: 4 in, 2 out]
              }
            }
          }
          event "Scope Reconnecting": Value Change {
            n454 = event-data() -> ()  [unwired: 1 in, 6 out]
            n455 = local read "Scope Connected"() -> (w788:bool)
            n456 = And(x=w788, y="Scope Reconnecting") -> (x .and. y?=w786:bool)
            n457 = case shown="True" w786 {
              tunnel: w785 -> [_ w802]
              frame False {
              }
              frame True {
                n458 = local read "Scope Address"() -> (w790:refnum<visa-resource-name>)
                n459 = call <vilib>:"Acquire Semaphore.vi"("semaphore"=w802) -> ("error out"=w791:errorcluster, "semaphore out"=w801:T6)  [unwired: 4 in, 1 out]
                n460 = property class="Instr"(reference=w790, error in=w791, "Timeout"=u32 2000 ("General Settings:Timeout Value")) -> (reference out=w793:refnum<visa-resource-name>, error out=w794:errorcluster)
                n461 = VISA Write(VISA resource name=w793, write buffer="*IDN?" ("ID query"), error in (no error)=w794) -> (VISA resource name out=w796:refnum<visa-resource-name>, error out=w797:errorcluster)  [unwired: 1 out]
                n462 = VISA Read(VISA resource name=w796, byte count=u32 1024, error in (no error)=w797) -> (error out=w789:errorcluster)  [unwired: 3 out]
                n463 = case shown="Error .." w789 {
                  selector: w789 -> [w803 w812]
                  tunnel: w801 -> [_ w811]
                  tunnel: [w803 w804] -> w800
                  frame No Error {
                  }
                  frame Error {
                    n464 = call <vilib>:"Clear Errors.vi"("error in (no error)"=w812) -> ("error out"=w810:errorcluster)  [unwired: 5 in, 1 out]
                    n465 = call <vilib>:"Release Semaphore.vi"("error in (no error)"=w810, "semaphore"=w811) -> ("error out"=w809:errorcluster)  [unwired: 4 in, 1 out]
                    n466 = property on="Disconnect Scope" class="Bool (strict)"(error in=w809, "Val(Sgnl)"=TRUE) -> (error out=w806:errorcluster)  [unwired: 1 in, 1 out]
                    n467 = property on="Measurements Running" class="Bool (strict)"(error in=w806) -> (error out=w805:errorcluster, "Value"=w807:bool)  [unwired: 1 in, 1 out]
                    n468 = case shown="True" w807 {
                      tunnel: w805 -> [w813 w818]
                      tunnel: [w813 w815] -> w804
                      frame False {
                      }
                      frame True {
                        n469 = call "Display Message to User"("error in (no error)"=w818, "Message"="Scope disconnected, stopping measurements.") -> ("error out"=w816:errorcluster)  [unwired: 8 in, 1 out]
                        n470 = property on="Stop Measurement" class="Bool (strict)"(error in=w816, "Val(Sgnl)"=TRUE) -> (error out=w815:errorcluster)  [unwired: 1 in, 1 out]
                      }
                    }
                  }
                }
                n471 = property on="Scope Reconnecting" class="Bool (strict)"(error in=w800, "Value"=FALSE) -> ()  [unwired: 1 in, 2 out]
              }
            }
          }
          event "Connect DMM", "Connect DMM 2": Value Change {
            n472 = event-data() -> ("CtlRef"=w840:refnum<vi>)  [unwired: 1 in, 5 out]
            n473 = call "Find Control Set from Control Reference.vi"("Control Set Array"=w828, "Control to Search For"=w840) -> ("error out"=w839:errorcluster, "Index"=w829:i32)  [unwired: 1 in]
            n474 = Index Array(array=w830, index=w829) -> (element=w819:T7)
            n475 = Unbundle By Name(w819) -> ("DMM Connected"=w827:refnum<vi>, "DMM Address"=w825:refnum<vi>, "DMM Model"=w822:refnum<vi>, "DMM Reset"=w823:refnum<vi>, "DMM Config on Startup"=w821:refnum<vi>, "Connect DMM"=w826:refnum<vi>, "Connected DMM"=w820:refnum<vi>, "Offline Controls"=w837:refnum<vi>[], "Online Controls"=w836:refnum<vi>[])  [unwired: 6 out]
            n476 = property class="Bool (strict)"(reference=w827, error in=w839) -> (reference out=w824:refnum<vi>, error out=w833:errorcluster, "Value"=w838:bool)
            n477 = property class="Bool (strict)"(reference=w826, error in=w833) -> (error out=w834:errorcluster, "Value"=w832:bool)  [unwired: 1 out]
            n478 = Not(x=w838) -> (.not. x?=w835:bool)
            n479 = And(x=w835, y=w832) -> (x .and. y?=w831:bool)
            n480 = case shown="True" w831 {
              tunnel: w834 -> [_ w852]
              tunnel: w837 -> [_ w842]
              tunnel: w836 -> [_ w870]
              tunnel: w830 -> [_ w854]
              tunnel: w829 -> [_ _]
              tunnel: w829 -> [_ _]
              tunnel: w825 -> [_ w848]
              tunnel: w824 -> [_ w847]
              tunnel: w823 -> [_ w846]
              tunnel: w822 -> [_ w845]
              tunnel: w821 -> [_ w844]
              tunnel: w820 -> [_ w843]
              tunnel: w819 -> [_ w841]
              frame False {
              }
              frame True {
                n481 = property class="VISAName"(reference=w848, error in=w852) -> (error out=w851:errorcluster, "Value"=w853:refnum<visa-resource-name>)  [unwired: 1 out]
                n482 = call "DMM Already Connected.vi"("error in (no error)"=w851, "Control Set Array"=w854, "DMM Address"=w853) -> ("error out"=w850:errorcluster, "Conflict Exists"=w849:bool)  [unwired: 1 in]
                n483 = case shown="False" w849 {
                  tunnel: w850 -> [w872 _]
                  tunnel: [w872 errorcluster {"status"=TRUE, "code"=-7999, "source"="Instrument already connected."} ("error constant")] -> w869
                  frame False {
                  }
                  frame True {
                  }
                }
                n484 = call "Set Control Visibility.vi"("error in"=w869, "Disabled"=T9."Disabled and Grayed Out", "Controls Reference Array"=w842) -> ("error out"=w858:errorcluster)  [unwired: 1 in]
                n485 = property class="Bool (strict)"(reference=w846, error in=w858) -> (error out=w857:errorcluster, "Value"=w864:bool)  [unwired: 1 out]
                n486 = property class="Ring (strict)"(reference=w845, error in=w857) -> (error out=w856:errorcluster, "Value"=w865:u16)  [unwired: 1 out]
                n487 = property class="Enum (strict)"(reference=w844, error in=w856) -> (error out=w855:errorcluster, "Value"=w863:enum16{"PC->DMM", "DMM->PC"})  [unwired: 1 out]
                n488 = call "Init DMM.vi"("DMM Reset"=w864, "DMM Control References Array"=w841, "error in"=w855, "DMM Config on Startup"=w863, "DMM Model"=w865, "DMM Address"=w853) -> ("error out"=w868:errorcluster, "Instrument Name"=w866:string, "VISA resource name out"=w867:refnum<visa-resource-name>)  [unwired: 1 in]
                n489 = case shown="No Error" w868 {
                  selector: w868 -> [w881 w887]
                  tunnel: [w882 "Not Connected"] -> w861
                  tunnel: w866 -> [w882 _]
                  tunnel: w867 -> [w880 _]
                  tunnel: w842 -> [_ w883]
                  tunnel: w870 -> [w874 _]
                  tunnel: [TRUE FALSE] -> w862
                  tunnel: [w875 w884] -> w860
                  frame No Error {
                    n490 = property class="Instr"(reference=w880, error in=w881, "Timeout"=-1) -> (error out=w877:errorcluster)  [unwired: 1 out]
                    n491 = call "Set Control Visibility.vi"("error in"=w877, "Disabled"=T9."Enabled", "Controls Reference Array"=w874) -> ("error out"=w875:errorcluster)  [unwired: 1 in]
                  }
                  frame Error {
                    n492 = Unbundle By Name(w887) -> ("source"=w888:string)
                    n493 = call <vilib>:"Clear Errors.vi"("error in (no error)"=w887) -> ("error out"=w886:errorcluster)  [unwired: 5 in, 1 out]
                    n494 = call "Display Message to User4"("error in (no error)"=w886, "Message"=w888) -> ("error out"=w885:errorcluster)  [unwired: 8 in, 1 out]
                    n495 = call "Set Control Visibility.vi"("error in"=w885, "Disabled"=T9."Enabled", "Controls Reference Array"=w883) -> ("error out"=w884:errorcluster)  [unwired: 1 in]
                  }
                }
                n496 = property class="Bool (strict)"(reference=w847, error in=w860, "Value"=w862) -> (error out=w859:errorcluster)  [unwired: 1 out]
                n497 = property class="Str"(reference=w843, error in=w859, "Value"=w861) -> ()  [unwired: 2 out]
              }
            }
          }
          event "Disconnect DMM", "Disconnect DMM 2": Value Change {
            n498 = event-data() -> ("CtlRef"=w911:refnum<vi>)  [unwired: 1 in, 5 out]
            n499 = call "Find Control Set from Control Reference.vi"("Control Set Array"=w897, "Control to Search For"=w911) -> ("error out"=w908:errorcluster, "Index"=w895:i32)  [unwired: 1 in]
            n500 = Index Array(array=w896, index=w895) -> (element=w894:T7)
            n501 = Unbundle By Name(w894) -> ("DMM Connected"=w893:refnum<vi>, "DMM Address"=w910:refnum<vi>, "DMM Model"=w909:refnum<vi>, "DMM Connected"=w907:refnum<vi>, "Connected DMM"=w906:refnum<vi>, "Disconnect DMM"=w892:refnum<vi>, "semaphore"=w905:T6, "Online Controls"=w903:refnum<vi>[], "Offline Controls"=w904:refnum<vi>[])  [unwired: 1 out]
            n502 = property class="Bool (strict)"(reference=w893, error in=w908) -> (error out=w902:errorcluster, "Value"=w899:bool)  [unwired: 1 out]
            n503 = property class="Bool (strict)"(reference=w892, error in=w902) -> (error out=w901:errorcluster, "Value"=w900:bool)  [unwired: 1 out]
            n504 = And(x=w899, y=w900) -> (x .and. y?=w898:bool)
            n505 = case shown="True" w898 {
              tunnel: [errorcluster {"status"=FALSE, "code"=0, "source"=""} ("error out") w932] -> _
              tunnel: w910 -> [_ w919]
              tunnel: w909 -> [_ w918]
              tunnel: w901 -> [_ w929]
              tunnel: w907 -> [_ w916]
              tunnel: w906 -> [_ w915]
              tunnel: w905 -> [_ w917]
              tunnel: w904 -> [_ w914]
              tunnel: w903 -> [_ w913]
              frame False {
              }
              frame True {
                n506 = property class="VISAName"(reference=w919, error in=w929) -> (error out=w928:errorcluster, "Value"=w927:refnum<visa-resource-name>)  [unwired: 1 out]
                n507 = property class="Ring (strict)"(reference=w918, error in=w928) -> (error out=w920:errorcluster, "Value"=w926:u16)  [unwired: 1 out]
                n508 = call <vilib>:"Acquire Semaphore.vi"("error in (no error)"=w920, "semaphore"=w917) -> ("error out"=w931:errorcluster, "semaphore out"=w935:T6)  [unwired: 3 in, 1 out]
                n509 = call "Disconnect DMM.vi"("error in"=w931, "DMM Model"=w926, "DMM Address"=w927) -> ("error out"=w930:errorcluster)  [unwired: 1 in]
                n510 = call "Set Control Visibility.vi"("error in"=w930, "Disabled"=T9."Enabled", "Controls Reference Array"=w914) -> ("error out"=w936:errorcluster)  [unwired: 1 in]
                n511 = call "Set Control Visibility.vi"("error in"=w936, "Disabled"=T9."Disabled and Grayed Out", "Controls Reference Array"=w913) -> ("error out"=w923:errorcluster)  [unwired: 1 in]
                n512 = property on="Property Node" class="Bool (strict)"(reference=w916, error in=w923, "Value"=FALSE) -> (error out=w922:errorcluster)  [unwired: 1 out]
                n513 = property on="Property Node" class="Str"(reference=w915, error in=w922, "Value"="Not Connected") -> (error out=w921:errorcluster)  [unwired: 1 out]
                n514 = call <vilib>:"Release Semaphore.vi"("error in (no error)"=w921, "semaphore"=w935) -> ("error out"=w932:errorcluster)  [unwired: 4 in, 1 out]
              }
            }
          }
          event "Identify DMM", "Identify DMM 2": Value Change {
            n515 = event-data() -> ("CtlRef"=w951:refnum<vi>)  [unwired: 1 in, 5 out]
            n516 = call "Find Control Set from Control Reference.vi"("Control Set Array"=w938, "Control to Search For"=w951) -> ("error out"=w948:errorcluster, "Index"=w940:i32)  [unwired: 1 in]
            n517 = Index Array(array=w939, index=w940) -> (element=w937:T7)
            n518 = Unbundle By Name(w937) -> ("DMM Connected"=w942:refnum<vi>, "DMM Address"=w950:refnum<vi>, "semaphore"=w949:T6, "Identify DMM"=w944:refnum<vi>)
            n519 = property class="Bool (strict)"(reference=w942, error in=w948) -> (error out=w943:errorcluster, "Value"=w947:bool)  [unwired: 1 out]
            n520 = property class="Bool (strict)"(reference=w944, error in=w943) -> (error out=w941:errorcluster, "Value"=w946:bool)  [unwired: 1 out]
            n521 = And(x=w947, y=w946) -> (x .and. y?=w945:bool)
            n522 = case shown="True" w945 {
              tunnel: w950 -> [_ w953]
              tunnel: w941 -> [_ w959]
              tunnel: w949 -> [_ w952]
              frame False {
              }
              frame True {
                n523 = property class="VISAName"(reference=w953, error in=w959) -> (error out=w957:errorcluster, "Value"=w958:refnum<visa-resource-name>)  [unwired: 1 out]
                n524 = call <vilib>:"Acquire Semaphore.vi"("error in (no error)"=w957, "semaphore"=w952) -> ("error out"=w956:errorcluster, "semaphore out"=w954:T6)  [unwired: 3 in, 1 out]
                n525 = VISA Write(VISA resource name=w958, write buffer="SYST:BEEP", error in (no error)=w956) -> (error out=w960:errorcluster)  [unwired: 2 out]
                n526 = call <vilib>:"General Error Handler.vi"("error in (no error)"=w960) -> ("error out"=w955:errorcluster)  [unwired: 10 in, 4 out]
                n527 = call <vilib>:"Release Semaphore.vi"("error in (no error)"=w955, "semaphore"=w954) -> ()  [unwired: 4 in, 2 out]
              }
            }
          }
          event "DMM Measurement Type", "DMM Measurement Type 2": Value Change {
            n528 = event-data() -> ("CtlRef"=w973:refnum<vi>)  [unwired: 1 in, 5 out]
            n529 = call "Find Control Set from Control Reference.vi"("Control Set Array"=w966, "Control to Search For"=w973) -> ("error out"=w974:errorcluster, "Index"=w965:i32)  [unwired: 1 in]
            n530 = Index Array(array=w967, index=w965) -> (element=w964:T7)
            n531 = Unbundle By Name(w964) -> ("DMM Connected"=w963:refnum<vi>, "DMM Address"=w971:refnum<vi>, "DMM Measurement Type"=w962:refnum<vi>, "DMM Model"=w969:refnum<vi>, "semaphore"=w968:T6)
            n532 = property class="Bool (strict)"(reference=w963, error in=w974) -> (error out=w970:errorcluster, "Value"=w972:bool)  [unwired: 1 out]
            n533 = case shown="True" w972 {
              tunnel: w971 -> [_ w978]
              tunnel: w962 -> [_ w977]
              tunnel: w970 -> [_ w983]
              tunnel: w969 -> [_ w976]
              tunnel: w968 -> [_ w975]
              frame False {
              }
              frame True {
                n534 = property class="VISAName"(reference=w978, error in=w983) -> (error out=w984:errorcluster, "Value"=w985:refnum<visa-resource-name>)  [unwired: 1 out]
                n535 = property class="Ring (strict)"(reference=w977, error in=w984) -> (error out=w982:errorcluster, "Value"=w979:i32)  [unwired: 1 out]
                n536 = property class="Ring (strict)"(reference=w976, error in=w982) -> (error out=w980:errorcluster, "Value"=w981:u16)  [unwired: 1 out]
                n537 = call <vilib>:"Acquire Semaphore.vi"("error in (no error)"=w980, "semaphore"=w975) -> ("error out"=w989:errorcluster, "semaphore out"=w991:T6)  [unwired: 3 in, 1 out]
                n538 = property class="Instr"(reference=w985, error in=w989, "Timeout"=-1) -> (reference out=w988:refnum<visa-resource-name>, error out=w987:errorcluster)
                n539 = call "Update DMM Settings.vi"("error in"=w987, "DMM Measurement Type"=w979, "DMM Model"=w981, "DMM Address"=w988) -> ("error out"=w986:errorcluster)  [unwired: 1 out]
                n540 = call <vilib>:"General Error Handler.vi"("error in (no error)"=w986) -> ("error out"=w992:errorcluster)  [unwired: 10 in, 4 out]
                n541 = call <vilib>:"Release Semaphore.vi"("error in (no error)"=w992, "semaphore"=w991) -> ()  [unwired: 4 in, 2 out]
              }
            }
          }
          event "DMM Reconnecting", "DMM Reconnecting 2": Value Change {
            n542 = event-data() -> ("CtlRef"=w1008:refnum<vi>)  [unwired: 1 in, 5 out]
            n543 = call "Find Control Set from Control Reference.vi"("Control Set Array"=w998, "Control to Search For"=w1008) -> ("error out"=w1009:errorcluster, "Index"=w997:i32)  [unwired: 1 in]
            n544 = Index Array(array=w999, index=w997) -> (element=w996:T7)
            n545 = Unbundle By Name(w996) -> ("DMM Connected"=w995:refnum<vi>, "DMM Reconnecting"=w993:refnum<vi>, "DMM Address"=w1004:refnum<vi>, "Disconnect DMM"=w994:refnum<vi>, "semaphore"=w1003:T6)
            n546 = property class="Bool (strict)"(reference=w995, error in=w1009) -> (error out=w1007:errorcluster, "Value"=w1006:bool)  [unwired: 1 out]
            n547 = property class="Bool (strict)"(reference=w993, error in=w1007) -> (error out=w1002:errorcluster, "Value"=w1005:bool)  [unwired: 1 out]
            n548 = And(x=w1006, y=w1005) -> (x .and. y?=w1010:bool)
            n549 = case shown="True" w1010 {
              tunnel: [_ w1025] -> w1000
              tunnel: w1004 -> [_ w1012]
              tunnel: w994 -> [_ w1014]
              tunnel: w1003 -> [_ w1011]
              tunnel: w1002 -> [_ w1013]
              frame False {
              }
              frame True {
                n550 = property class="VISAName"(reference=w1012, error in=w1013) -> ("Value"=w1015:refnum<visa-resource-name>)  [unwired: 2 out]
                n551 = call <vilib>:"Acquire Semaphore.vi"("semaphore"=w1011) -> ("error out"=w1017:errorcluster, "semaphore out"=w1026:T6)  [unwired: 4 in, 1 out]
                n552 = property class="Instr"(reference=w1015, error in=w1017, "Timeout"=u32 2000 ("General Settings:Timeout Value")) -> (reference out=w1019:refnum<visa-resource-name>, error out=w1020:errorcluster)
                n553 = VISA Write(VISA resource name=w1019, write buffer="*IDN?" ("ID query"), error in (no error)=w1020) -> (VISA resource name out=w1022:refnum<visa-resource-name>, error out=w1023:errorcluster)  [unwired: 1 out]
                n554 = VISA Read(VISA resource name=w1022, byte count=u32 1024, error in (no error)=w1023) -> (error out=w1016:errorcluster)  [unwired: 3 out]
                n555 = case shown="Error .." w1016 {
                  selector: w1016 -> [w1029 w1039]
                  tunnel: [w1027 w1034] -> w1025
                  tunnel: w1026 -> [w1028 w1038]
                  tunnel: w1014 -> [_ w1030]
                  frame No Error {
                    n556 = call <vilib>:"Release Semaphore.vi"("error in (no error)"=w1029, "semaphore"=w1028) -> ("error out"=w1027:errorcluster)  [unwired: 4 in, 1 out]
                  }
                  frame Error {
                    n557 = call <vilib>:"Clear Errors.vi"("error in (no error)"=w1039) -> ("error out"=w1037:errorcluster)  [unwired: 5 in, 1 out]
                    n558 = call <vilib>:"Release Semaphore.vi"("error in (no error)"=w1037, "semaphore"=w1038) -> ("error out"=w1032:errorcluster)  [unwired: 4 in, 1 out]
                    n559 = property on="Property Node" class="Bool (strict)"(reference=w1030, error in=w1032, "Val(Sgnl)"=TRUE) -> (error out=w1031:errorcluster)  [unwired: 1 out]
                    n560 = property on="Measurements Running" class="Bool (strict)"(error in=w1031) -> (error out=w1036:errorcluster, "Value"=w1035:bool)  [unwired: 1 in, 1 out]
                    n561 = case shown="True" w1035 {
                      tunnel: w1036 -> [w1040 w1045]
                      tunnel: [w1040 w1041] -> w1034
                      frame False {
                      }
                      frame True {
                        n562 = call "Display Message to User3"("error in (no error)"=w1045, "Message"="DMM disconnected, stopping measurements.") -> ("error out"=w1042:errorcluster)  [unwired: 8 in, 1 out]
                        n563 = property on="Stop Measurement" class="Bool (strict)"(error in=w1042, "Val(Sgnl)"=TRUE) -> (error out=w1041:errorcluster)  [unwired: 1 in, 1 out]
                      }
                    }
                  }
                }
              }
            }
            n564 = property on="Property Node" class="Bool (strict)"(reference=w993, error in=w1000, "Value"=FALSE) -> ()  [unwired: 2 out]
          }
          event "Start Measurement": Value Change {
            n565 = event-data() -> ()  [unwired: 1 in, 6 out]
            n566 = local read "Measurements Running"() -> (w1052:bool)
            n567 = local read "Scope Connected"() -> (w1050:bool)
            n568 = Not(x=w1052) -> (.not. x?=w1049:bool)
            n569 = Compound Arithmetic op=AND("Start Measurement", w1050, w1049) -> (w1048:bool)
            n570 = case shown="True" w1048 {
              tunnel: w1053 -> [_ w1082]
              tunnel: [_ FALSE] -> w1047
              tunnel: w1046 -> [_ w1054]
              frame False {
              }
              frame True {
                n571 = local write "Traces Saved"(0) -> ()
                n572 = Build Array("Trace Number", "Timestamp", "Time (s)", "Voltage (V)") -> (w1074:string[])
                n573 = property on="PS Connected" class="Bool (strict)"() -> ("Value"=w1079:bool)  [unwired: 2 in, 2 out]
                n574 = case shown="True" w1079 {
                  tunnel: w1074 -> [w1133 w1138]
                  tunnel: [w1133 w1134] -> w1061
                  frame False {
                  }
                  frame True {
                    n575 = Insert Into Array(array=w1138, new element="Diode Power Supply Voltage (V)") -> (w1135:string[])  [unwired: 1 in]
                    n576 = Insert Into Array(array=w1135, new element="Diode Power Supply Current (A)") -> (w1134:string[])  [unwired: 1 in]
                  }
                }
                n577 = local read "PS Connected 2"() -> (w1059:bool)
                n578 = case shown="True" w1059 {
                  tunnel: w1061 -> [w1092 w1097]
                  tunnel: [w1092 w1093] -> w1060
                  frame False {
                  }
                  frame True {
                    n579 = Insert Into Array(array=w1097, new element="Amp Power Supply Voltage (V)") -> (w1094:string[])  [unwired: 1 in]
                    n580 = Insert Into Array(array=w1094, new element="Amp Power Supply Current (A)") -> (w1093:string[])  [unwired: 1 in]
                  }
                }
                n581 = property on="DMM Connected" class="Bool (strict)"() -> ("Value"=w1073:bool)  [unwired: 2 in, 2 out]
                n582 = case shown="True" w1073 {
                  tunnel: w1060 -> [w1125 w1128]
                  tunnel: [w1125 w1126] -> w1063
                  frame False {
                  }
                  frame True {
                    n583 = property on="DMM Measurement Type" class="Ring (strict)"() -> ("Value"=w1130:i32, "Strings []"=w1131:string[])  [unwired: 2 in, 2 out]
                    n584 = Index Array(array=w1131, index=w1130) -> (element=w1129:string)
                    n585 = Concatenate Strings("DMM " ("string"), w1129) -> (w1127:string)
                    n586 = Insert Into Array(array=w1128, new element=w1127) -> (w1126:string[])  [unwired: 1 in]
                  }
                }
                n587 = case shown="\"Store Average/Std. Dev. for each Point\"" "Measurement Mode" {
                  tunnel: [_ errorcluster {"status"=TRUE, "code"=-8000, "source"="Mode not implemented yet."} ("error constant")] -> w1068
                  frame "Store All Traces in Single File", Default {
                  }
                  frame "Store Average/Std. Dev. for each Point" {
                    n588 = Build Array("Timestamp", "Time (s)", "Avg. Voltage (V)", "Std. Dev. (V)") -> ()  [unwired: 1 out]
                  }
                }
                n589 = local read "DMM Connected 2"() -> (w1064:bool)
                n590 = case shown="True" w1064 {
                  tunnel: w1063 -> [w1098 w1100]
                  tunnel: [w1098 w1099] -> w1062
                  frame False {
                  }
                  frame True {
                    n591 = property on="DMM Measurement Type 2" class="Ring (strict)"() -> ("Value"=w1104:i32, "Strings []"=w1105:string[])  [unwired: 2 in, 2 out]
                    n592 = Index Array(array=w1105, index=w1104) -> (element=w1102:string)
                    n593 = Concatenate Strings("DMM 2 " ("string"), w1102) -> (w1101:string)
                    n594 = Insert Into Array(array=w1100, new element=w1101) -> (w1099:string[])  [unwired: 1 in]
                  }
                }
                "Headers" <- w1062
                n595 = call "Set Control Visibility.vi"("error in"=w1068, "Disabled"=T9."Disabled and Grayed Out", "Controls Reference Array"=w1082) -> ("error out"=w1080:errorcluster)  [unwired: 1 in]
                n596 = call "File Dialog"("error in"=w1080) -> ("selected path"=w1072:path, "error out"=w1089:errorcluster)  [unwired: 11 in, 2 out]
                n597 = call <vilib>:"Get File Extension.vi"("file"=w1072) -> ("filename without extension"=w1066:string, "lowercase file extension"=w1071:string, "dup file"=w1065:path)  [unwired: 6 in, 2 out]
                n598 = Equal?(x=w1071, y="csv") -> (x = y?=w1069:bool)
                n599 = case shown="True" w1069 {
                  tunnel: [w1120 w1124] -> w1090
                  tunnel: w1072 -> [w1119 _]
                  tunnel: w1065 -> [_ w1124]
                  frame False {
                    n600 = Path To String(path=w1119) -> (string=w1123:string)
                    n601 = Concatenate Strings(w1123, ".csv") -> (w1121:string)
                    n602 = String To Path(string=w1121) -> (path=w1120:path)
                  }
                  frame True {
                  }
                }
                n603 = Build Array("Delimiter") -> (w1057:u8[])
                n604 = Type Cast(type="", x=w1057) -> (*(type *) &x=w1055:string)
                n605 = case shown="\"Store All Traces in Single File\", Default" "Measurement Mode" {
                  tunnel: [w1112 w1113] -> w1091
                  tunnel: w1090 -> [w1110 _]
                  tunnel: w1089 -> [w1109 w1118]
                  tunnel: [w1108 w1118] -> w1083
                  tunnel: w1062 -> [w1107 _]
                  tunnel: w1066 -> [_ w1115]
                  tunnel: w1065 -> [_ w1117]
                  tunnel: w1055 -> [w1106 _]
                  frame "Store All Traces in Single File", Default {
                    n606 = call-poly <vilib>:"Write Delimited Spreadsheet.vi"("file path (dialog if empty)"=w1110, "1D data"=w1107, "append to file? (new file:F)"=FALSE, "error in (no error)"=w1109, "delimiter (\\t)"=w1106) -> ("error out"=w1108:errorcluster)  [unwired: 9 in, 1 out]
                    n607 = Strip Path(path=w1110) -> (name=w1112:string)  [unwired: 1 out]
                  }
                  frame "Store All Traces in Separate Files" {
                    n608 = Strip Path(path=w1117) -> (stripped path=w1116:path)  [unwired: 1 out]
                    n609 = Build Path(base path=w1116, name or relative path=w1115) -> (appended path=w1114:path)
                    n610 = Path To String(path=w1114) -> (string=w1113:string)
                  }
                }
                "Filename" <- w1091
                n611 = case shown="No Error" w1083 {
                  selector: w1083 -> [w1141 w1148]
                  tunnel: w1090 -> [w1147 _]
                  tunnel: [w1146 w1148] -> w1088
                  tunnel: w1082 -> [w1144 w1149]
                  tunnel: T9."Disabled and Grayed Out" ("Disabled") -> [w1143 _]
                  tunnel: T9."Enabled" ("Disabled") -> [w1142 w1150]
                  tunnel: w1054 -> [w1139 _]
                  frame No Error {
                    n612 = call "Set Control Visibility.vi"("error in"=w1141, "Disabled"=w1143, "Controls Reference Array"=w1144) -> ("error out"=w1145:errorcluster)  [unwired: 1 in]
                    n613 = call "Set Control Visibility.vi"("error in"=w1145, "Disabled"=w1142, "Controls Reference Array"=w1139) -> ("error out"=w1146:errorcluster)  [unwired: 1 in]
                    "Full File Path" <- w1147
                    "Measurements Running" <- TRUE
                  }
                  frame Error {
                    n614 = call "Set Control Visibility.vi"("Disabled"=w1150, "Controls Reference Array"=w1149) -> ()  [unwired: 2 in, 1 out]
                  }
                }
                n615 = call <vilib>:"General Error Handler.vi"("error in (no error)"=w1088) -> ()  [unwired: 10 in, 5 out]
              }
            }
            n616 = local write "Start Measurement"(w1047) -> ()
          }
          event "Stop Measurement": Value Change {
            n617 = event-data() -> ()  [unwired: 1 in, 6 out]
            n618 = local read "Measurements Running"() -> (w1163:bool)
            n619 = local read "Scope Connected"() -> (w1158:bool)
            n620 = Compound Arithmetic op=AND("Stop Measurement", w1163, w1158) -> (w1161:bool)
            n621 = case shown="True" w1161 {
              tunnel: w1160 -> [_ w1169]
              tunnel: [_ w1165] -> w1159
              tunnel: w1156 -> [_ w1164]
              frame False {
              }
              frame True {
                n622 = local write "Measurements Running"(FALSE) -> ()
                n623 = call "Set Control Visibility.vi"("Disabled"=T9."Enabled", "Controls Reference Array"=w1169) -> ("error out"=w1170:errorcluster)  [unwired: 2 in]
                n624 = call "Set Control Visibility.vi"("error in"=w1170, "Disabled"=T9."Disabled and Grayed Out", "Controls Reference Array"=w1164) -> ("error out"=w1165:errorcluster)  [unwired: 1 in]
              }
            }
            n625 = property on="Stop Measurement" class="Bool (strict)"(error in=w1159, "Value"=FALSE) -> ()  [unwired: 1 in, 2 out]
          }
          event "Exit": Value Change {
            n626 = event-data() -> ()  [unwired: 1 in, 5 out]
            n627 = local read "Scope Connected"() -> (w1213:bool)
            n628 = case shown="True" w1213 {
              tunnel: [_ w1216] -> w1210
              frame False {
              }
              frame True {
                n629 = property on="Disconnect Scope" class="Bool (strict)"("Val(Sgnl)"=FALSE) -> (error out=w1216:errorcluster)  [unwired: 2 in, 1 out]
              }
            }
            n630 = local read "PS Connected"() -> (w1211:bool)
            n631 = case shown="True" w1211 {
              tunnel: w1210 -> [_ w1215]
              frame False {
              }
              frame True {
                n632 = property on="Disconnect PS" class="Bool (strict)"(error in=w1215, "Value"=FALSE) -> ()  [unwired: 1 in, 2 out]
              }
            }
            n633 = local read "Power Supply Config on Startup"() -> (w1174:enum16{"PC->Power Supply", "Power Supply->PC"})
            n634 = local read "DMM Measurement Type"() -> (w1202:i32)
            n635 = local read "Scope Config on Startup"() -> (w1189:enum16{"PC->Scope", "Scope->PC"})
            n636 = local read "Horizontle Trace Display"() -> (w1197:i32)
            n637 = local read "DMM Config on Startup"() -> (w1175:enum16{"PC->DMM", "DMM->PC"})
            n638 = local read "Record Sample Length"() -> (w1193:i32)
            n639 = local read "Power Supply Address"() -> (w1194:refnum<visa-resource-name>)
            n640 = local read "Power Supply Model"() -> (w1171:T3)
            n641 = local read "Measurement Mode"() -> (w1195:T4)
            n642 = local read "Waveform Source"() -> (w1178:u16)
            n643 = local read "Input Impedance"() -> (w1196:u16)
            n644 = local read "Traces to Acquire"() -> (w1188:u64)
            n645 = local read "Trigger Coupling"() -> (w1187:i32)
            n646 = local read "ResetPS Settings"() -> (w1191:bool)
            n647 = local read "Repetitive Signal"() -> (w1173:bool)
            n648 = local read "Horizontle Scale"() -> (w1198:i32)
            n649 = local read "Trigger Level (V)"() -> (w1186:dbl)
            n650 = local read "Scope Address"() -> (w1190:refnum<visa-resource-name>)
            n651 = local read "Trigger Source"() -> (w1184:u16)
            n652 = local read "DMM Address"() -> (w1203:refnum<visa-resource-name>)
            n653 = local read "Reset Settings"() -> (w1192:bool)
            n654 = local read "Current Limit"() -> (w1205:dbl)
            n655 = local read "Voltage Level"() -> (w1180:sgl)
            n656 = local read "Voltage Limit"() -> (w1179:dbl)
            n657 = local read "Trigger Slope"() -> (w1185:i32)
            n658 = local read "Vertical Scale"() -> (w1181:u16)
            n659 = local read "Scope Model"() -> (w1176:u16)
            n660 = local read "DMM Model"() -> (w1201:u16)
            n661 = local read "Trigger Type"() -> (w1183:u16)
            n662 = local read "Current Trip"() -> (w1204:dbl)
            n663 = local read "DMM Reset"() -> (w1200:bool)
            n664 = local read "Filter Mode"() -> (w1199:u16)
            n665 = local read "Bandwidth"() -> (w1208:u16)
            n666 = local read "Trip Mode"() -> (w1182:u16)
            n667 = local read "Coupling"() -> (w1206:u16)
            n668 = Bundle By Name(cluster=T10 {"Bandwidth"=0, "Coupling"=0, "Current Limit"=0.0, "Current Trip"=0.0, "DMM Address"="", "DMM Measurement Type"=0, "DMM Model"=0, "DMM Reset"=FALSE, "Filter Mode"=0, "Horizontle Scale"=0, "Horizontle Trace Display"=0, "Input Impedance"=0, "Power Supply Address"="", "Record Sample Length"=0, "Reset Settings"=FALSE, "ResetPS Settings"=FALSE, "Scope Address"="", "Scope Config on Startup"=0, "Traces to Acquire"=0, "Trigger Coupling"=0, "Trigger Level (V)"=0.0, "Trigger Slope"=0, "Trigger Source"=0, "Trigger Type"=0, "Trip Mode"=0, "Vertical Scale"=0, "Voltage Level"=0.0, "Voltage Limit"=0.0, "Waveform Source"=0, "Scope Model"=1, "DMM Config on Startup"=enum."DMM->PC", "Power Supply Config on Startup"=enum."Power Supply->PC", "Repetitive Signal"=FALSE, "Measurement Mode"=enum."Store All Traces in Single File", "Power Supply Model"=enum."Keithley 248"} ("output cluster"), "Bandwidth"=w1208, "Coupling"=w1206, "Current Limit"=w1205, "Current Trip"=w1204, "DMM Address"=w1203, "DMM Measurement Type"=w1202, "DMM Model"=w1201, "DMM Reset"=w1200, "Filter Mode"=w1199, "Horizontle Scale"=w1198, "Horizontle Trace Display"=w1197, "Input Impedance"=w1196, "Measurement Mode"=w1195, "Power Supply Address"=w1194, "Power Supply Model"=w1171, "Record Sample Length"=w1193, "Reset Settings"=w1192, "ResetPS Settings"=w1191, "Scope Address"=w1190, "Scope Config on Startup"=w1189, "Traces to Acquire"=w1188, "Trigger Coupling"=w1187, "Trigger Level (V)"=w1186, "Trigger Slope"=w1185, "Trigger Source"=w1184, "Trigger Type"=w1183, "Trip Mode"=w1182, "Vertical Scale"=w1181, "Voltage Level"=w1180, "Voltage Limit"=w1179, "Waveform Source"=w1178, "Scope Model"=w1176, "DMM Config on Startup"=w1175, "Power Supply Config on Startup"=w1174, "Repetitive Signal"=w1173) -> (w1177:T10)
          }
        }
      }
      n669 = Current VI's Path() -> (path=w220:path)
      n670 = call "Save Settings To XML File.vi"("error in (no error)"=w221, "Settings File Name"="config.xml", "Settings File Path"=w220) -> ("error out"=w223:errorcluster)  [unwired: 2 in]
      n671 = call <vilib>:"Clear Errors.vi"("error in (no error)"=w223) -> ("error out"=w222:errorcluster)  [unwired: 5 in, 1 out]
    }
    frame Error {
      n672 = call <vilib>:"General Error Handler.vi"("error in (no error)"=w1218) -> ()  [unwired: 10 in, 5 out]
    }
  }
